vi "AODScanner1.vi"() -> ()   [LabVIEW 2014]
uses:
  AODAcq/AODAcq.lvclass
  <vilib>/DAQmx/write.llb/DAQmx Write (Analog DBL 1Chan 1Samp).vi
  Motion Stabilization/GlobalVars.vi
  <vilib>/Utility/error.llb/Error Cluster From Error Code.vi
  <vilib>/rvi/errors/niLvFpgaAdjustHostInterfaceError.vi
  <vilib>/DAQmx/read.llb/DAQmx Read (Analog Wfm 1Chan NSamp).vi
  <vilib>/rvi/interface/nirviMethod/nirviMethod.xnode
  FPGA_Control/AODRef.ctl
  FPGA Bitfiles/AodScanner_FPGATarget_AODControl(FPGA)_TyJc9yYmyGA.lvbitx
  <vilib>/rvi/interface/nirviReadWriteControl/nirviReadWriteControl.xnode
  <vilib>/FPGAPlugInAG/PXIe-7965R/niLvFpga_ReadFifo_PXIe-7965R.vi
  <vilib>/rvi/errors/niLvFpgaMergeErrorWithErrorCode.vi
  NiFpgaLv.dll
panel:
  out "globals_semaphore":T1
  out "Scan Settings Saved":T2
  out "y_scale":dbl
  out "x_scale":dbl
  out "Motion Points (Ch1)":u32
  in  "Per Cell Motion Analysis":bool
  in  "Sampling Structure":u16(ring) items=["Cube Vertices"]
  out "EventDone":bool
  in  "ForcePointScan":bool
  out "Selection":u32
  in  "ForceVolumeScan":bool
  out "Scan Settings (um) Saved":T2={"XStart"=-100, "XEnd"=100, "XNum"=250, "YStart"=-100, "YEnd"=100, "YNum"=250, "ZStart"=-30, "ZEnd"=70, "ZNum"=60}
  out "Motion FIFO":refnum<queue>
  out "Points_um":dbl[][](array[numeric])
  out "Stopped":bool
  in  "Power":dbl(slide)=2.5 min=0.0 max=5.0 step=0.1 scale=0.0..2.5
  in  "Debug":bool
  out "Number of Motion Planes":i32
  out "Motion Plane Centers":i32[][](array[numeric])
  in  "GridPoints":u16=10
  out "X-Y Motion Points":i32[][](array[numeric])
  out "Y-Z Motion Points":i32[][](array[numeric])
  out "error out":errorcluster
  out "error out 2":errorcluster
  in  "External Magnification":dbl=1.3
  in  "Matlab Server IP Address":string="10.21.16.18"
  in  "Matlab Server Shared Folder":string="c:\\temp"
  out "Histogram":dynamicdata(graph)
  out "ROIs":T3(array[cluster])
  out "Motion ROIs":T3(array[cluster])
  out "Waveform Chart":waveform(dbl)(graph)
  out "Ephys":bool
  in  "Points":i32[][](array[numeric])
  in  "Abort":bool
  out "ScanProgress":dbl(slide) scale=0.0..1.0
  in  "Simulated Motion Signal":bool
  in  "TraceElements":u32=10000
  out "Out Points":i32[][](array[numeric])
  in  "Tab Control":enum32{"Setup", "Volume", "Traces", "Motion"}(tab)
  in  "Motor Refractory Time":dbl=2.0
  in  "Motor Correction Threshold":dbl=2.0 format="%#_13g"
  in  "Motion Tracking":bool
  in  "Auto Recentering":bool
  in  "XNum":i32=100
  in  "YNum":i32=100
  in  "Onset (fraction)":dbl=0.99 format="%#_13g"
  in  "Offset (fraction)":dbl=0.01 format="%#_13g"
  in  "Post Recentering Wait (ms)":u32=1000
  in  "Store Raw":bool
  in  "Disp Volume":bool=TRUE
  in  "Save Volume":bool
  in  "Ephys Acq":bool
  in  "Motion rate (Hz)":dbl=10.0
  in  "Scan Settings (um)":T2={"XStart"=-100, "XEnd"=100, "XNum"=250, "YStart"=-100, "YEnd"=100, "YNum"=250, "ZStart"=-30, "ZEnd"=70, "ZNum"=60}
  in  "Objective":enum16{"20x Olympus"}(ring)
  in  "Scan Time (s)":dbl=300.0
  in  "Volume Reps":i32=1 min=1 max=10000
  in  "Volume Scan":bool
  in  "Points Scan":bool
  in  "Motion Channel To Analyze":i32=2 min=1 max=2
  in  "Motion Analysis":bool
  in  "Auto Motion Plane Params":T4={"Z Offset Per Box (um)"=3, "Box Size (um)"=16.0}
  in  "Mirror Ch1 Display":bool
  in  "ClearMotionCenters":bool
  in  "Point Centering":bool=TRUE
  in  "Recenter":bool caption="OK Button"
  out "Cells Selected":u32
  in  "Contrast":dbl(slide)=99.63636363636364 scale=98.0..100.0
  out "ImCh2":T5(plugin-control)
  out "ImCh1":T5(plugin-control)
  in  "Section":dbl min=0.0 max=59.0 step=1.0
  in  "Segment":bool
  out "Motion Increment":u32
  in  "Offset":dbl(slide)=0.010101010101010102 scale=0.0..1.0
  in  "ClearPoints":bool
  out "Total Motion Points":i32
  out "Number of Motion Volumes":i32
  out "Motion Ch1":T5(plugin-control)
  out "Ephys Signals":waveform(dbl)[](graph)
  in  "Baseline Offset":dbl
  in  "Decimate":bool
  in  "Spacing":dbl=100.0
  out "Traces":waveform(dbl)[](graph)
  in  "Down Rate":i32=500
  out "Motion Detection Error":bool
  in  "Enable Calibration":bool
  in  "Analyze Nth Frames":i32=1 min=1 step=1
  out "Elements in Data Queue":i32
  out "Out of Limits":bool
  in  "Position Shift Limit (Microns)":dbl=3.0 min=0.0
  out "Z1":waveform(dbl)(graph)
  out "Y1":waveform(dbl)(graph)
  out "X1":waveform(dbl)(graph)
  out "VolData":i32[][](array[numeric])
  out "Progress":dbl(slide) scale=0.0..1.0
  out "Scan Settings":T2
  in  "VolumeElements":u32=10000
  out "Recording File":path
  out "Objective Position":cluster{"X":dbl, "Y":dbl, "Z":dbl}
  out "Lens Magnification":i32=20
  out "Finished":bool
  out "Image samples remaining":u32
  out "Motion samples remaining":u32
  out "Temporal samples remaining":u32
  out "Raw samples remaining":u32
  in  "stop":bool
  out "AODAcq out":refnum<class "AODAcq.lvclass">
  out "Volume":bool
  out "Scan":bool
  in  "SweepSettings":bool
  out "Numeric":i32=299
  # "On"
  # "Off"
  # "sec"
  # "um"
  # "Motor"
  # "AOD+Motor"
  # "Off"
  # "On"
  # "Volume Resolution (points)"
  # "Behavior Pause"
  # "Off"
  # "On"
  # "Off"
  # "On"
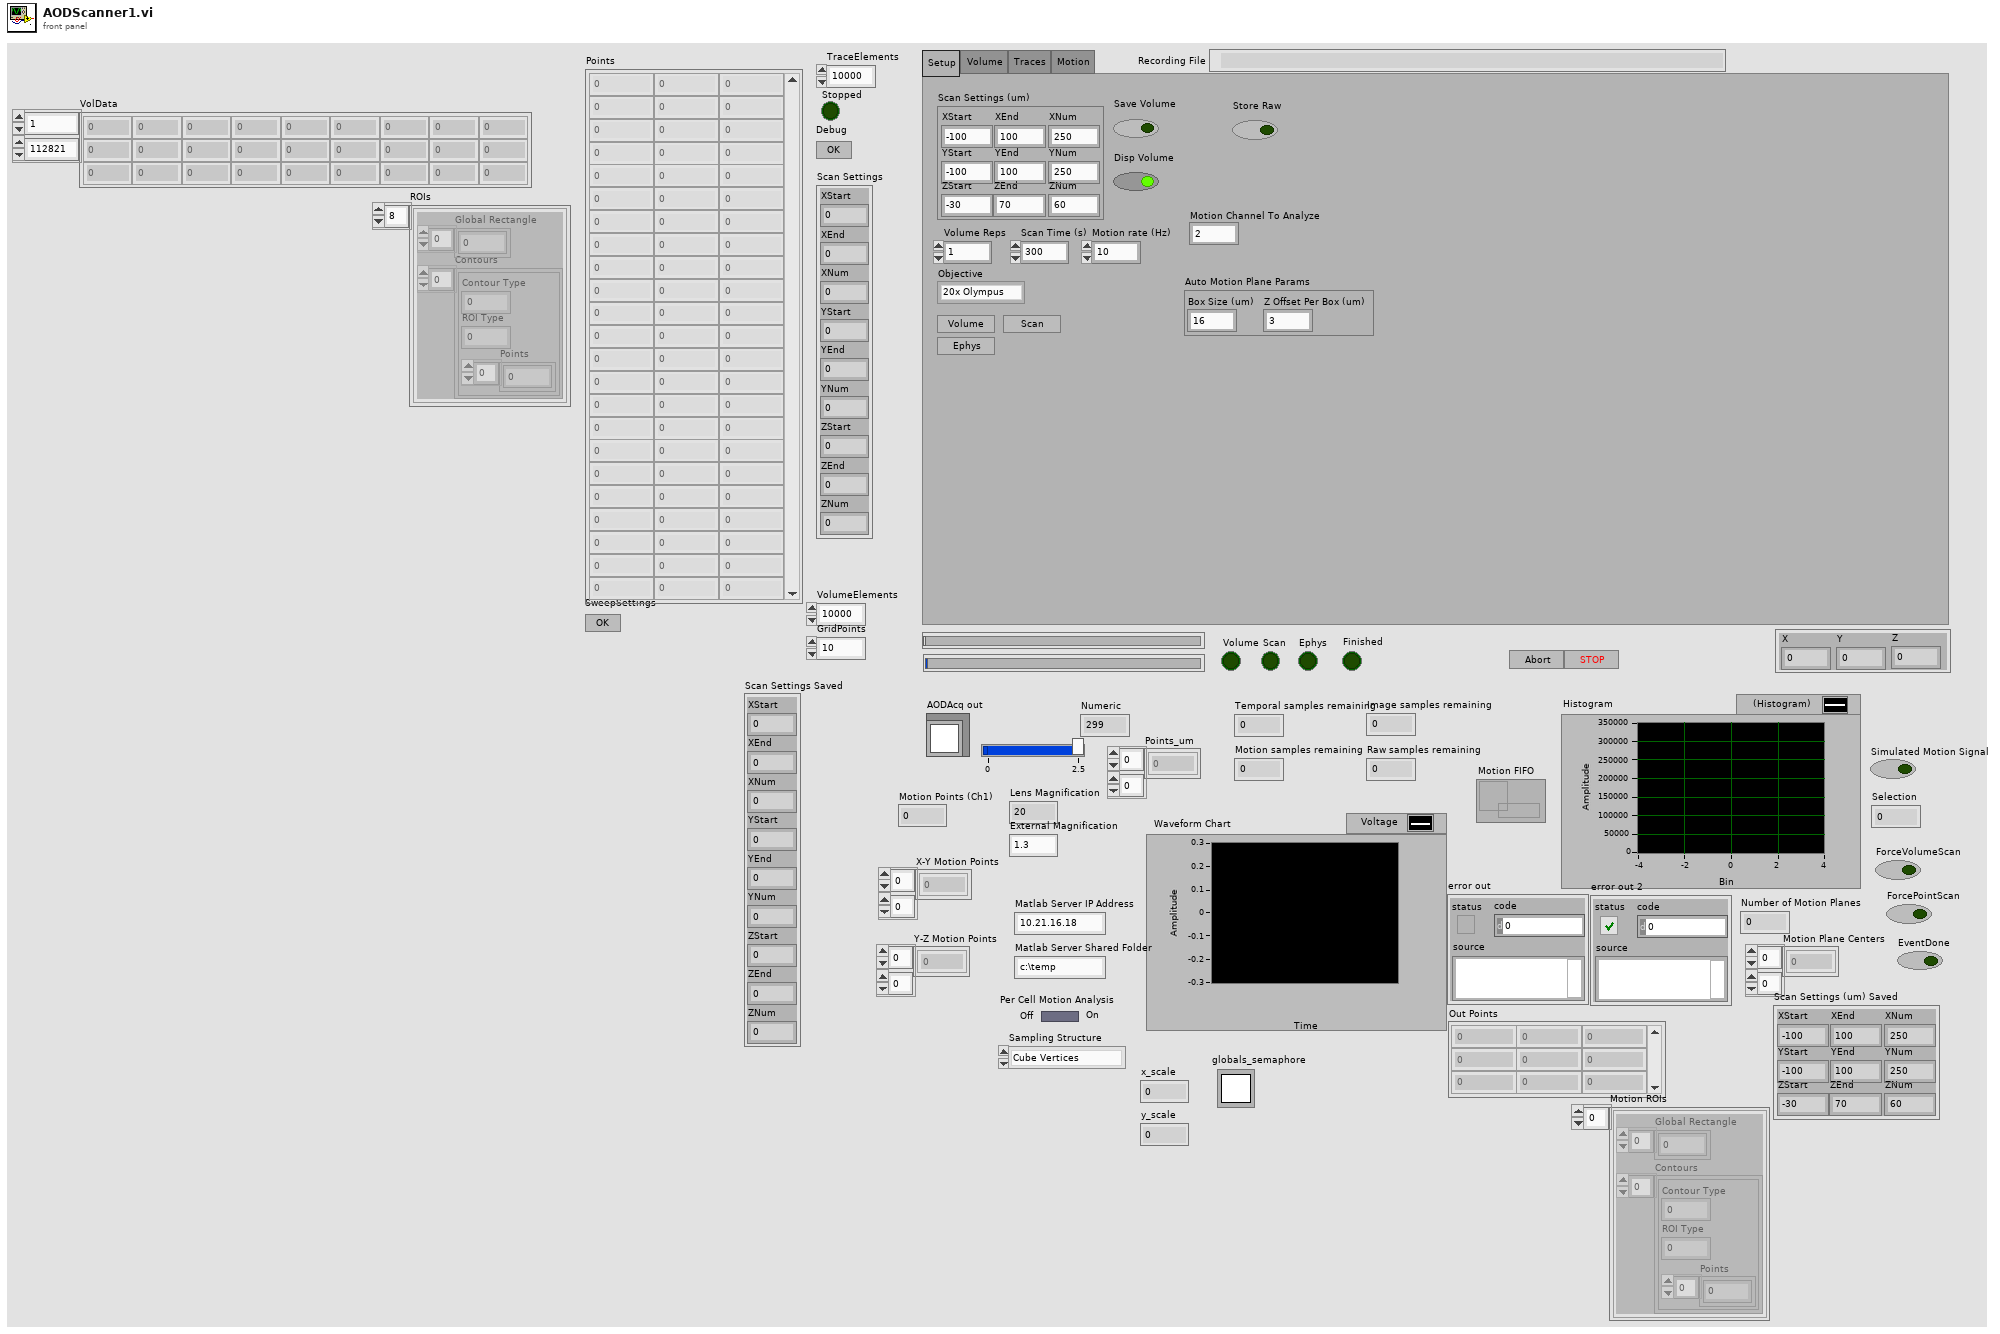
[diagram p1: front panel]
types:
  T1 = typedef "Semaphore RefNum" = refnum<k1>
  T2 = cluster{"XStart":i32, "XEnd":i32, "XNum":i32, "YStart":i32, "YEnd":i32, "YNum":i32, "ZStart":i32, "ZEnd":i32, "ZNum":i32}
  T3 = cluster{"Global Rectangle":i32[], "Contours":cluster{"Contour Type":u32, "ROI Type":u32, "Points":i32[]}[]}[]
  T4 = cluster{"Z Offset Per Box (um)":i32, "Box Size (um)":dbl}
  T5 = typedef "IMAQ Image.ctl" = refnum<image>
  T6 = cluster{"gridsize":u16, "data":i32[][], "coordinates":i32[][], "settings":i32[], "settings_um":i32[], "needsreference":bool}
  T7 = typedef "Image Type" = u32
  T8 = cluster{"Global Rectangle":i32[], "Contours":cluster{"Contour Type":u32, "ROI Type":u32, "Points":i32[]}[]}
  T9 = cluster{"queue out":refnum<queue>, "queue out":refnum<queue>, "queue out":refnum<queue>, "queue out":refnum<queue>}
  T10 = cluster{"Restarted":bool, "Enable Calibration":bool, "Position Shift Limit (Microns)":dbl, "Frame Num":dbl, "Sampling Interval":dbl, "Analyze Nth Frames":i32}
  T11 = typedef "AODRef.ctl" = refnum<k20>
  T12 = cluster{"X":waveform(dbl), "Y":waveform(dbl), "Z":waveform(dbl), "Out of Limits":bool, "Motion Detection Error":bool, "Flush Queue":i32, "Movement Signal":dbl[], "Movement Detection Time":dbl}
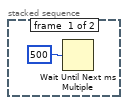
[diagram p2: hidden frame]
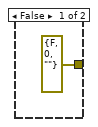
[diagram p4: hidden frame]
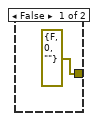
[diagram p5: hidden frame]
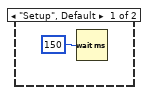
[diagram p6: hidden frame]
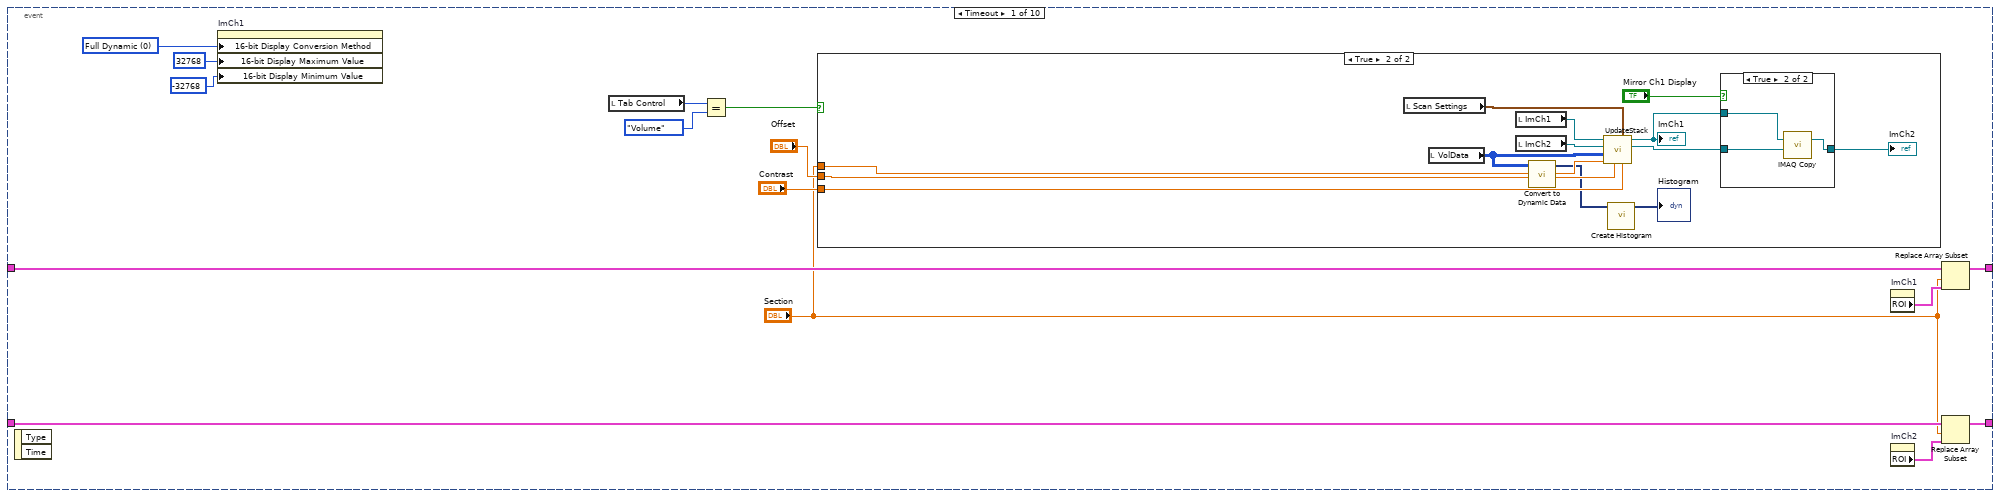
[diagram p8: hidden frame]
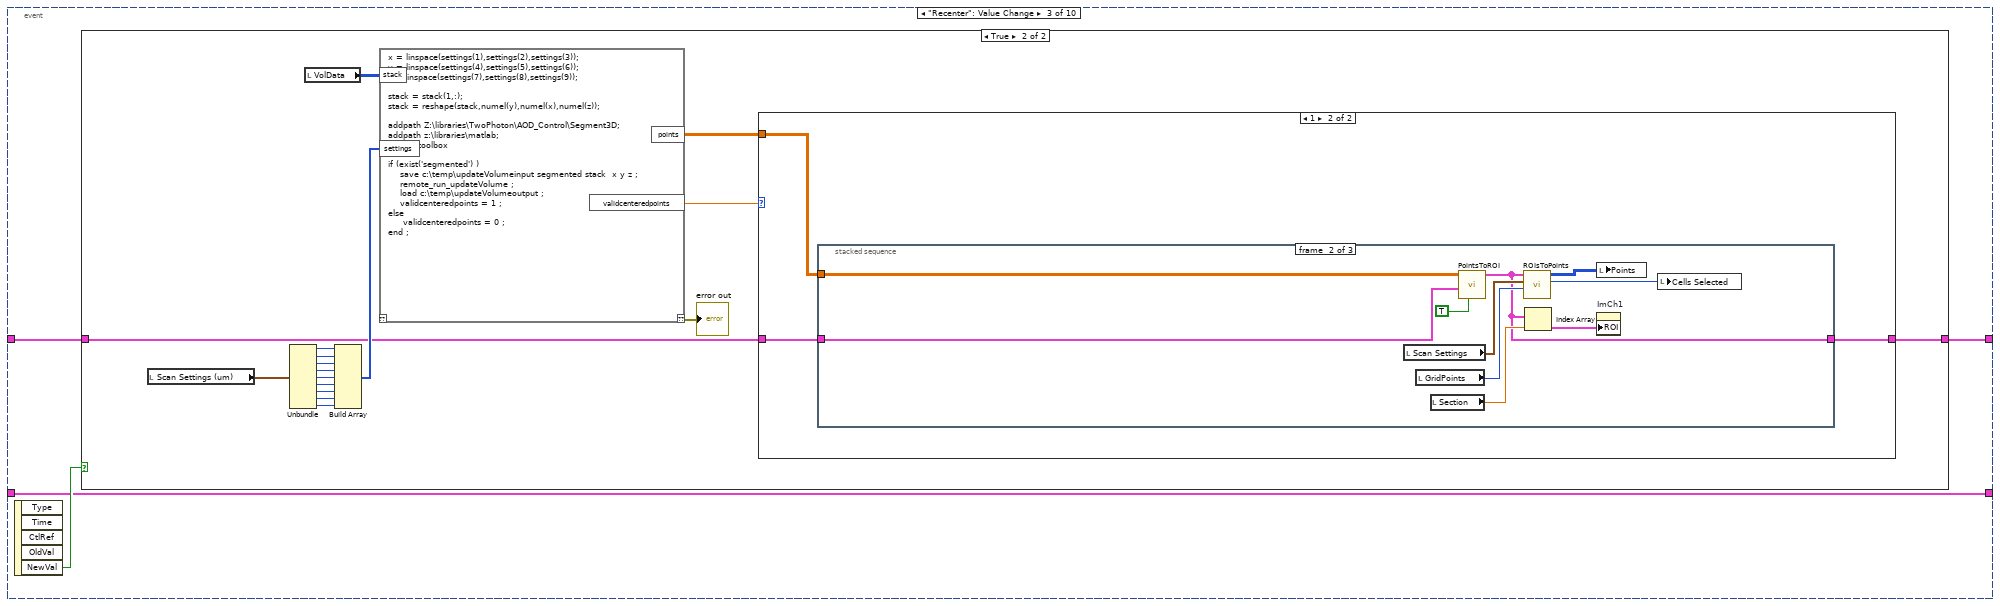
[diagram p12: hidden frame]
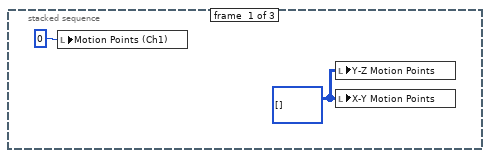
[diagram p15: hidden frame]
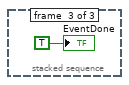
[diagram p16: hidden frame]
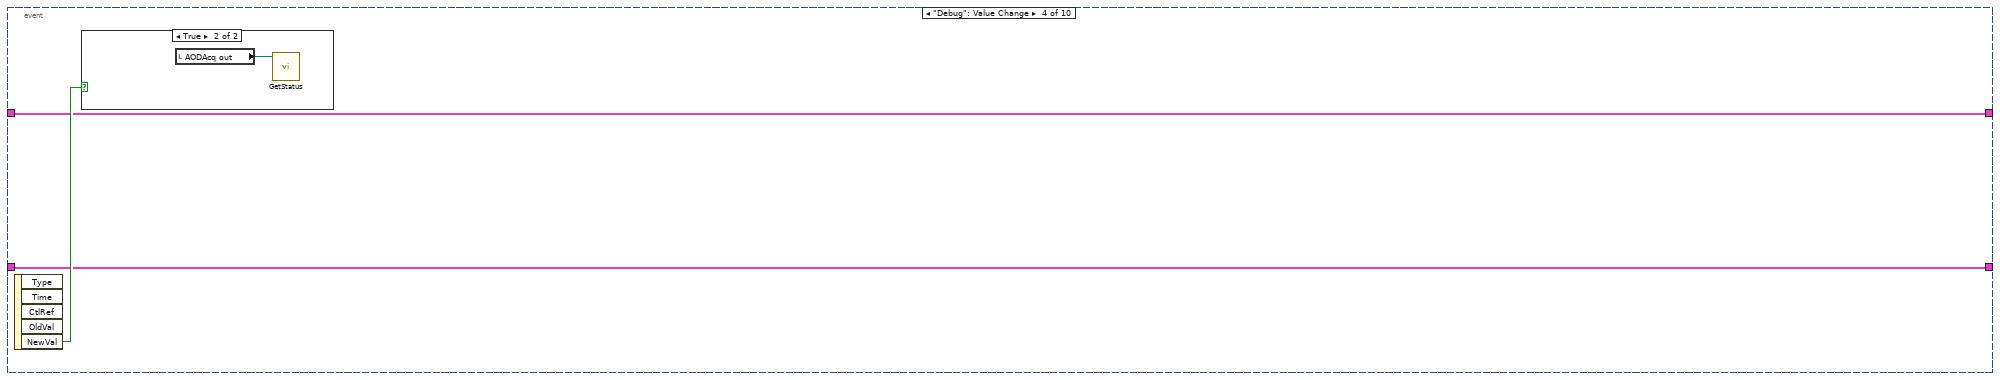
[diagram p17: hidden frame]
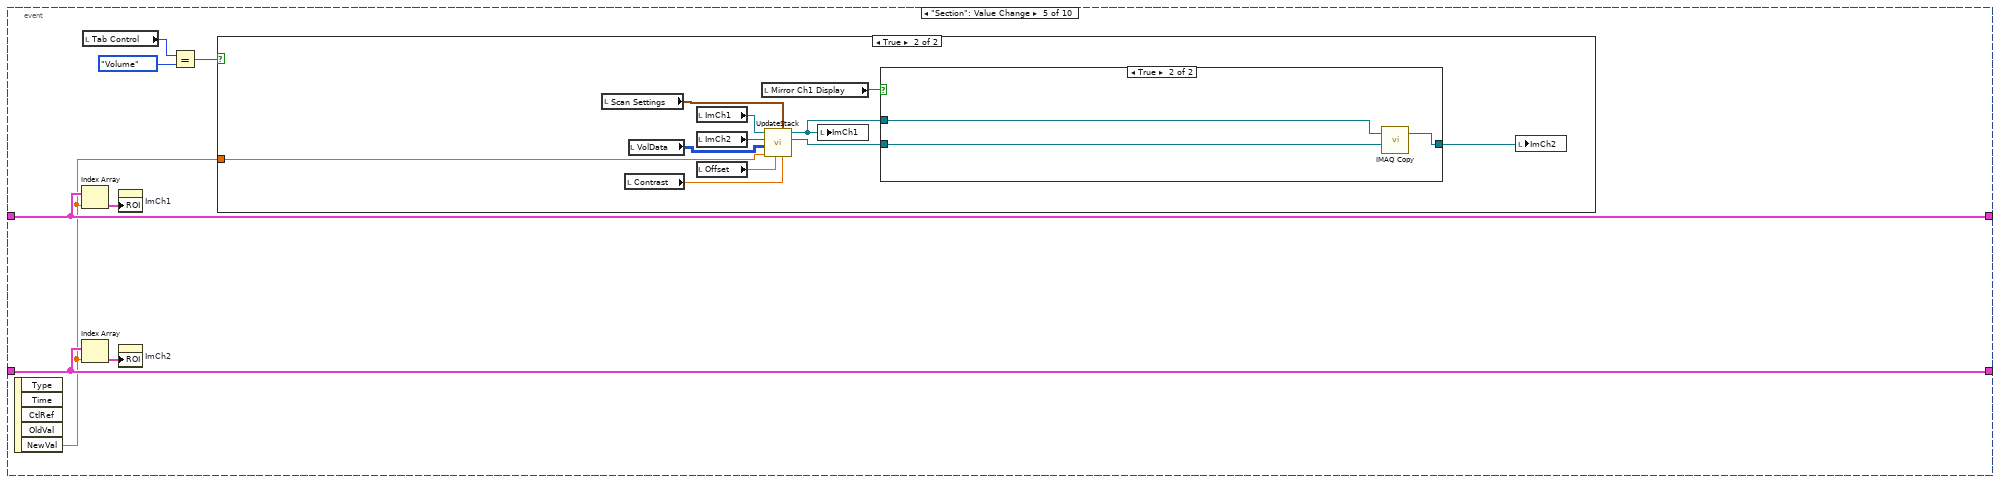
[diagram p19: hidden frame]
diagram:
  w7 = FALSE ("ForceVolumeScan")
  w24 = 100 ("max queue size (-1, unlimited)")
  w29 = T7 2 items=["Grayscale (U8)", "Grayscale (I16)", "Grayscale (SGL)", "Complex (CSG)", "RGB (U32)", "HSL (U32)", "RGB (U64)", "Grayscale (U16)"] ("Image Type")
  w5 = waveform(i32)[] []
  w39 = T7 0 items=["Grayscale (U8)", "Grayscale (I16)", "Grayscale (SGL)", "Complex (CSG)", "RGB (U32)", "HSL (U32)", "RGB (U64)", "Grayscale (U16)"] ("Image Type")
  w15 = T8 {"Global Rectangle"=[], "Contours"=[]} ("ROI")
  w49 = refnum<k21> "AOD Gain"  # DAQmx Global Channel
  n1 = local read "Scan Settings (um)"() -> (w43:T2)
  n2 = local write "ForceVolumeScan"(w7) -> ()
  n3 = local write "ForcePointScan"(w7) -> ()
  n4 = local write "Stopped"(FALSE ("Stopped")) -> ()
  n5 = local write "Stopped"(FALSE ("Stopped")) -> ()
  n6 = global write "GlobalVars.vi" "VI Open"(FALSE ("VI Open")) -> ()
  n7 = local write "Tab Control"(enum32{"Setup", "Volume", "Traces", "Motion"}."Setup" ("Tab Control")) -> ()
  n8 = Reciprocal(x="Motion rate (Hz)") -> (1/x=w17:dbl)
  n9 = global write "GlobalVars.vi" "Sampling Interval (sec)"(w17) -> ()
  n10 = call <vilib>:"DAQmx Create Task.vi"("global virtual channels"=w49) -> ("task out"=w48:refnum<k21>, "error out"=w47:errorcluster)  [unwired: 4 in, 9 out]
  n11 = call "IMAQ Create"("Image Name"="Im1", "Image Type"=w39) -> ("New Image"=w51:T5)  [unwired: 3 in, 1 out]
  n12 = call "IMAQ Create"("Image Name"="Im2", "Image Type"=w39) -> ("New Image"=w50:T5)  [unwired: 3 in, 1 out]
  n13 = Unbundle By Name(w43) -> ("ZNum"=w14:i32)
  n14 = call "IMAQ Create"("Image Name"="Mot1", "Image Type"=w29) -> ("New Image"=→"Motion Ch1":T5)  [unwired: 3 in, 1 out]
  n15 = while {
    tunnel: w48 -> [w60]
    tunnel: w47 -> [w59]
    tunnel: [w58] -> w46
    tunnel: [w57] -> w45
    stop <- w56 stop-if-true
    n16 = Wait (ms)(milliseconds to wait=u32 1000) -> ()  [unwired: 1 out]
    n17 = local read "Stopped"() -> (w56:bool)
    n18 = call-poly <vilib>:"DAQmx Write.vi"("task/channels in"=w60, "data"="Power", "error in"=w59) -> ("task out"=w58:refnum<k21>, "error out"=w57:errorcluster)  [unwired: 10 in, 1 out]
  }
  n19 = local write "ImCh1"(w51) -> ()
  n20 = local write "ImCh2"(w50) -> ()
  n21 = Obtain Queue(max queue size (-1, unlimited)=w24, element data type=waveform(i32)[] []) -> (queue out=w35:refnum<queue>)  [unwired: 3 in, 2 out]
  n22 = Obtain Queue(max queue size (-1, unlimited)=w24, element data type=waveform(dbl)[] []) -> (queue out=w36:refnum<queue>)  [unwired: 3 in, 2 out]
  n23 = Obtain Queue(max queue size (-1, unlimited)=w24, element data type=w5) -> (queue out=w34:refnum<queue>)  [unwired: 3 in, 2 out]
  n24 = Obtain Queue(element data type=w5) -> (queue out=w4:refnum<queue>)  [unwired: 4 in, 2 out]
  n25 = call <vilib>:"Obtain Semaphore Reference.vi"("name (unnamed)"="globals") -> ("error out"=w1:errorcluster, "semaphore"=w2:T1)  [unwired: 4 in, 1 out]
  "globals_semaphore" <- w2
  n26 = Obtain Queue(name (unnamed)="Motion FIFO", element data type=0) -> (queue out=w10:refnum<queue>)  [unwired: 3 in, 2 out]
  "Motion FIFO" <- w10
  n27 = Obtain Queue(max queue size (-1, unlimited)=100, name (unnamed)="MotionAnalysis", element data type=T6 {"gridsize"=0, "data"=[], "coordinates"=[], "settings"=[], "settings_um"=[], "needsreference"=FALSE}) -> (queue out=w8:refnum<queue>)  [unwired: 2 in, 2 out]
  n28 = Decrement(x=w14) -> (x-1=w38:i32)
  n29 = Initialize Array(w15, w14) -> (w42:T3)
  n30 = Initialize Array(w15, w14) -> (w13:T3)
  n31 = while {
    shift-right: [w63] -> _
    shift-left: w42 -> [w67]
    shift-right: [w62] -> _
    shift-left: w13 -> [w64]
    stop <- w65 stop-if-true
    n32 = event shown="[1] \"Segment\": Value Change" {
      selector: _ -> [_ _ _ _ _ _ _ _ _ _]
      dyn-events: _ -> [_ _ _ _ _ _ _ _ _ _]
      timeout: 200 -> [_ _ _ _ _ _ _ _ _ _]
      tunnel: w67 -> [w81 w102 w142 w181 w190 w218 w219 w232 w236 w248]
      tunnel: [w82 w101 w143 w181 w190 w215 w219 w231 w237 w248] -> w63
      tunnel: [w69 w100 w141 w180 w185 w207 w220 w228 w235 w249] -> w62
      tunnel: w64 -> [w72 w100 w141 w180 w185 w207 w225 w230 w235 w247]
      event Timeout {
        w77 = u32 0 items=["Full Dynamic", "Downshift", "Given Range", "90% Dynamic", "Given Percent Range"] ("16-bit Display Mapping:Conversion Method")
        n33 = event-data() -> ()  [unwired: 1 in, 2 out]
        n34 = property on="ImCh1" class="ImageControl"("16-bit Display Conversion Method"=w77, "16-bit Display Maximum Value"=32768 ("16-bit Display Mapping:Maximum Value"), "16-bit Display Minimum Value"=-32768 ("16-bit Display Mapping:Maximum Value")) -> ()  [unwired: 2 in, 2 out]
        n35 = local read "Tab Control"() -> (w79:enum32{"Setup", "Volume", "Traces", "Motion"})
        n36 = Equal?(x=w79, y=enum32{"Setup", "Volume", "Traces"}."Volume") -> (x = y?=w68:bool)
        n37 = case shown="True" w68 {
          tunnel: "Section" -> [_ w92]
          tunnel: "Offset" -> [_ w91]
          tunnel: "Contrast" -> [_ w90]
          frame False {
          }
          frame True {
            n38 = local read "Scan Settings"() -> (w93:T2)
            n39 = local read "VolData"() -> (w89:i32[][])
            n40 = local read "ImCh1"() -> (w95:T5)
            n41 = local read "ImCh2"() -> (w94:T5)
            n42 = call "Convert to Dynamic Data"("2D Array"=w89) -> ("Dynamic Data Type"=w88:dynamicdata)  [unwired: 3 in]
            n43 = call "UpdateStack.vi"("Contrast"=w90, "Scan Settings"=w93, "Offset"=w91, "Section"=w92, "ImData"=w89, "Im2 2"=w94, "Im1 In"=w95) -> ("Im2 Out"=w83:T5, "Im1 Out"=w85:T5)  [unwired: 3 in]
            "ImCh1" <- w85
            n44 = call "Create Histogram"("Signal"=w88) -> ("Histogram"=→"Histogram":dynamicdata)  [unwired: 9 in, 1 out]
            n45 = case shown="True" "Mirror Ch1 Display" {
              tunnel: w85 -> [_ w98]
              tunnel: [w96 w97] -> w84
              tunnel: w83 -> [w96 w99]
              frame False {
              }
              frame True {
                n46 = call "IMAQ Copy"("Image Dst"=w99, "Image Src"=w98) -> ("Image Dst Out"=w97:T5)  [unwired: 4 in, 1 out]
              }
            }
            "ImCh2" <- w84
          }
        }
        n47 = property on="ImCh1" class="ImageControl"() -> ("ROI"=w80:T8)  [unwired: 2 in, 2 out]
        n48 = property on="ImCh2" class="ImageControl"() -> ("ROI"=w71:T8)  [unwired: 2 in, 2 out]
        n49 = Replace Array Subset(array=w81, new element=w80, index="Section") -> (w82:T3)
        n50 = Replace Array Subset(array=w72, new element=w71, index="Section") -> (w69:T3)
      }
      event "Segment": Value Change {
        n51 = event-data() -> ("NewVal"=w103:bool)  [unwired: 1 in, 4 out]
        n52 = case shown="True" w103 {
          tunnel: w102 -> [w104 w122]
          tunnel: [w104 w126] -> w101
          frame False {
          }
          frame True {
            n53 = local read "Scan Settings (um)"() -> (w140:T2)
            n54 = local read "Lens Magnification"() -> (w118:i32)
            n55 = local read "Scan Settings (um)"() -> (w120:T2)
            n56 = Boolean To (0,1)(Boolean="Point Centering") -> (0, 1=w123:i16)
            n57 = Unbundle(w140) -> ("XStart"=w139:i32, "XEnd"=w138:i32, "XNum"=w137:i32, "YStart"=w136:i32, "YEnd"=w135:i32, "YNum"=w134:i32, "ZStart"=w133:i32, "ZEnd"=w132:i32, "ZNum"=w131:i32)
            n58 = Build Array(w139, w138, w137, w136, w135, w134, w133, w132, w131) -> (w112:i32[])
            n59 = To Double Precision Float(number=w123) -> (double precision float=w116:dbl)
            n60 = local read "VolData"() -> (w130:i32[][])
            n61 = Concatenate Strings("Matlab Server IP Address", "," ("string"), "Matlab Server Shared Folder") -> (w107:string)
            n62 = call "ROIsToSelCells.vi"("Scan Settings"=w120, "ROI"=w122) -> ("Points_um"=w119:dbl[][])  [unwired: 8 in, 1 out]
            n63 = Build Array (concatenate)(w118, "External Magnification", w116, w112) -> (w111:dbl[])
            n64 = script code="if (feature('numcores')>1)\n     if (~matlabpool('size') > 0)\n         matlabpool(min(feature('numcores'),12)) ;\n     end ;\nend ;\n\nlens = params(1) ;\nmagnification = params(2) ;\nenablecentering = params(3) ;\nsettings = params(4:end) ;\n\ncomma = strfind(textparams, ',') ;\nip = textparams(1:comma-1) ;\nsharedfolder = textparams(comma+1:end) ;\n\nx = linspace(settings(1),settings(2),settings(3));\ny = linspace(settings(4),settings(5),settings(6));\nz = linspace(settings(7),settings(8),settings(9));\n\nvol = vol(1,:);\nvol = reshape(vol,numel(y),numel(x),numel(z));\n\nrehash toolbox\nserver_ip = ip ;\nserver_shareddir = sharedfolder ;\n%save c:\\temp\\serverinfo server_ip ;\n\n%save c:\\temp\\segmenterinput vol x y z points lens magnification ip sharedfolder enablecentering ;\n%remote_run_segmenter ;\nseg = aod.Segmenter(vol, x, y, z, points, lens, magnification, ip, sharedfolder, enablecentering ) ;\nsegmented = SegmenterDisplay(seg) ;\n\nfilename = sprintf('%s\\\\seg.mat', sharedfolder) ;\nload(filename) ;\npoints = centered_coordinates;\npositions = points; % in microns\n\n% Need to convert points into indicies into the array\nfor i = 1:size(points,1)\n   [~,idx] = min(abs(points(i,1)-x)); points(i,1) = idx;\n   [~,idx] = min(abs(points(i,2)-y)); points(i,2) = idx;\n   [~,idx] = min(abs(points(i,3)-z)); points(i,3) = idx;\nend\noutpoints = points ;"("vol"=w130, "params"=w111, "textparams"=w107, "points"=w119) -> ("??"=→"error out 2":errorcluster, "outpoints"=w106:dbl[][], "positions"=w105:dbl[][])  [unwired: 1 in]
            n65 = call "PointsToROI.vi"("Old ROIs"=w122, "Points"=w106) -> ("ROIs"=w126:T3)  [unwired: 9 in]
            n66 = local write "Points_um"(w105) -> ()
            n67 = local read "Scan Settings"() -> (w128:T2)
            n68 = local read "GridPoints"() -> (w121:u16)
            n69 = local read "Section"() -> (w125:dbl)
            n70 = Index Array(array=w126, index=w125) -> (element=w127:T8)
            n71 = call "ROIsToPoints.vi"("GridPoints"=w121, "Scan Settings"=w128, "ROI"=w126) -> ("Number of motion points"=w109:i32, "Number of points"=w129:i32, "Points"=w108:i32[][])  [unwired: 4 in, 2 out]
            n72 = local write "Points"(w108) -> ()
            n73 = property on="ImCh1" class="ImageControl"("ROI"=w127) -> ()  [unwired: 2 in, 2 out]
            n74 = local write "Cells Selected"(w129) -> ()
            n75 = local write "Motion Points (Ch1)"(w109) -> ()
          }
        }
      }
      event "Recenter": Value Change {
        n76 = event-data() -> ("NewVal"=w144:bool)  [unwired: 1 in, 4 out]
        n77 = case shown="True" w144 {
          tunnel: [w145 w148] -> w143
          tunnel: w142 -> [w145 w149]
          frame False {
          }
          frame True {
            n78 = local read "Scan Settings (um)"() -> (w150:T2)
            n79 = Unbundle(w150) -> ("XStart"=w162:i32, "XEnd"=w161:i32, "XNum"=w160:i32, "YStart"=w159:i32, "YEnd"=w158:i32, "YNum"=w157:i32, "ZStart"=w156:i32, "ZEnd"=w155:i32, "ZNum"=w154:i32)
            n80 = local read "VolData"() -> (w152:i32[][])
            n81 = Build Array(w162, w161, w160, w159, w158, w157, w156, w155, w154) -> (w153:i32[])
            n82 = script code="x = linspace(settings(1),settings(2),settings(3));\ny = linspace(settings(4),settings(5),settings(6));\nz = linspace(settings(7),settings(8),settings(9));\n\nstack = stack(1,:);\nstack = reshape(stack,numel(y),numel(x),numel(z));\n\naddpath Z:\\libraries\\TwoPhoton\\AOD_Control\\Segment3D;\naddpath z:\\libraries\\matlab;\nrehash toolbox\n\nif (exist('segmented') )\n    save c:\\temp\\updateVolumeinput segmented stack  x y z ;\n    remote_run_updateVolume ;\n    load c:\\temp\\updateVolumeoutput ;\n    validcenteredpoints = 1 ;\nelse\n     validcenteredpoints = 0 ;\nend ;"("stack"=w152, "settings"=w153) -> ("??"=→"error out":errorcluster, "points"=w151:dbl[][], "validcenteredpoints"=w147:dbl)  [unwired: 1 in]
            n83 = case shown="1" w147 {
              tunnel: w151 -> [_ w166]
              tunnel: w149 -> [w163 w165]
              tunnel: [w163 w164] -> w148
              frame 0, Default {
              }
              frame 1 {
                n84 = stacked-sequence {
                  tunnel: w166 -> [_ w178 _]
                  tunnel: w165 -> [_ w174 _]
                  tunnel: [_ w171 _] -> w164
                  frame #0 {
                    w167 = i32[][] [] ("Points")
                    n85 = local write "Motion Points (Ch1)"(u32 0 ("Number of Motion Points")) -> ()
                    n86 = local write "Y-Z Motion Points"(w167) -> ()
                    n87 = local write "X-Y Motion Points"(w167) -> ()
                  }
                  frame #1 {
                    n88 = local read "Scan Settings"() -> (w175:T2)
                    n89 = local read "GridPoints"() -> (w176:u16)
                    n90 = local read "Section"() -> (w172:dbl)
                    n91 = call "PointsToROI.vi"("Clear Motion Planes"=TRUE, "Old ROIs"=w174, "Points"=w178) -> ("ROIs"=w171:T3)  [unwired: 8 in]
                    n92 = call "ROIsToPoints.vi"("GridPoints"=w176, "Scan Settings"=w175, "ROI"=w171) -> ("Number of points"=w177:i32, "Points"=w170:i32[][])  [unwired: 4 in, 3 out]
                    n93 = Index Array(array=w171, index=w172) -> (element=w173:T8)
                    n94 = local write "Points"(w170) -> ()
                    n95 = property on="ImCh1" class="ImageControl"("ROI"=w173) -> ()  [unwired: 2 in, 2 out]
                    n96 = local write "Cells Selected"(w177) -> ()
                  }
                  frame #2 {
                    "EventDone" <- TRUE ("EventDone")
                  }
                }
              }
            }
          }
        }
      }
      event "Debug": Value Change {
        n97 = event-data() -> ("NewVal"=w182:bool)  [unwired: 1 in, 4 out]
        n98 = case shown="True" w182 {
          frame False {
          }
          frame True {
            n99 = local read "AODAcq out"() -> (w183:refnum<class "AODAcq.lvclass">)
            n100 = call-dynamic "GetStatus.vi"("AODAcq in"=w183) -> ()  [unwired: 8 in, 3 out]
          }
        }
      }
      event "Section": Value Change {
        n101 = event-data() -> ("NewVal"=w184:dbl)  [unwired: 1 in, 4 out]
        n102 = Index Array(array=w190, index=w184) -> (element=w191:T8)
        n103 = Index Array(array=w185, index=w184) -> (element=w186:T8)
        n104 = local read "Tab Control"() -> (w189:enum32{"Setup", "Volume", "Traces", "Motion"})
        n105 = property on="ImCh1" class="ImageControl"("ROI"=w191) -> ()  [unwired: 2 in, 2 out]
        n106 = property on="ImCh2" class="ImageControl"("ROI"=w186) -> ()  [unwired: 2 in, 2 out]
        n107 = Equal?(x=w189, y=enum32{"Setup", "Volume", "Traces"}."Volume") -> (x = y?=w187:bool)
        n108 = case shown="True" w187 {
          tunnel: w184 -> [_ w199]
          frame False {
          }
          frame True {
            n109 = local read "Scan Settings"() -> (w198:T2)
            n110 = local read "Contrast"() -> (w196:dbl)
            n111 = local read "VolData"() -> (w202:i32[][])
            n112 = local read "ImCh1"() -> (w200:T5)
            n113 = local read "ImCh2"() -> (w201:T5)
            n114 = local read "Offset"() -> (w197:dbl)
            n115 = local read "Mirror Ch1 Display"() -> (w192:bool)
            n116 = call "UpdateStack.vi"("Contrast"=w196, "Scan Settings"=w198, "Offset"=w197, "Section"=w199, "ImData"=w202, "Im2 2"=w201, "Im1 In"=w200) -> ("Im2 Out"=w194:T5, "Im1 Out"=w195:T5)  [unwired: 3 in]
            n117 = local write "ImCh1"(w195) -> ()
            n118 = case shown="True" w192 {
              tunnel: w195 -> [_ w205]
              tunnel: [w203 w204] -> w193
              tunnel: w194 -> [w203 w206]
              frame False {
              }
              frame True {
                n119 = call "IMAQ Copy"("Image Dst"=w206, "Image Src"=w205) -> ("Image Dst Out"=w204:T5)  [unwired: 4 in, 1 out]
              }
            }
            n120 = local write "ImCh2"(w193) -> ()
          }
        }
      }
      event "GridPoints": Value Change; "ImCh1": Mouse Up {
        n121 = event-data() -> ()  [unwired: 1 in, 3 out]
        n122 = local read "Section"() -> (w216:dbl)
        n123 = local read "Scan Settings"() -> (w214:T2)
        n124 = property on="ImCh1" class="ImageControl"() -> ("ROI"=w217:T8)  [unwired: 2 in, 2 out]
        n125 = Replace Array Subset(array=w218, new element=w217, index=w216) -> (w215:T3)
        n126 = call "ROIsToPoints.vi"("GridPoints"="GridPoints", "Scan Settings"=w214, "ROI"=w215) -> ("X-Y Motion Points"=→"X-Y Motion Points":i32[][], "Number of motion points"=→"Motion Points (Ch1)":i32, "Number of points"=→"Cells Selected":i32, "Points"=w212:i32[][], "Y-Z Motion Points"=→"Y-Z Motion Points":i32[][])  [unwired: 4 in]
        n127 = local write "Points"(w212) -> ()
      }
      event "ImCh2": Mouse Up {
        n128 = event-data() -> ()  [unwired: 1 in, 3 out]
        n129 = local read "Section"() -> (w226:dbl)
        n130 = local read "Scan Settings"() -> (w224:T2)
        n131 = property on="ImCh2" class="ImageControl"() -> ("ROI"=w227:T8)  [unwired: 2 in, 2 out]
        n132 = local read "GridPoints"() -> (w223:u16)
        n133 = Replace Array Subset(array=w225, new element=w227, index=w226) -> (w220:T3)
        n134 = call "ROIsToPoints.vi"("GridPoints"=w223, "Scan Settings"=w224, "ROI"=w220) -> ("Number of points"=→"Number of Motion Planes":i32, "Points"=→"Motion Plane Centers":i32[][])  [unwired: 4 in, 3 out]
      }
      event "Scan Settings (um).ZNum": Value Change {
        n135 = event-data() -> ("NewVal"=w229:i32)  [unwired: 1 in, 4 out]
        n136 = Decrement(x=w229) -> (x-1=w233:i32)
        n137 = property on="Section" class="DigNum (strict)"("Maximum"=w233, "Minimum"=0.0 ("Data Entry Limits:Minimum")) -> ()  [unwired: 2 in, 2 out]
        n138 = Reshape Array(w232, w229) -> (w231:T3)
        n139 = Reshape Array(w230, w229) -> (w228:T3)
      }
      event "ClearPoints": Value Change {
        n140 = event-data() -> ("NewVal"=w238:bool)  [unwired: 1 in, 4 out]
        n141 = case shown="True" w238 {
          tunnel: [w239 w246] -> w237
          tunnel: w236 -> [w239 _]
          frame False {
          }
          frame True {
            w240 = u32 0 ("Number of Motion Points")
            w241 = i32[][] [] ("Points")
            w245 = T8 {"Global Rectangle"=[], "Contours"=[]} ("ROI")
            n142 = local write "Points"(w241) -> ()
            n143 = local write "Points_um"(dbl[][] [] ("Points_um")) -> ()
            n144 = local write "Cells Selected"(w240) -> ()
            n145 = local write "Motion Points (Ch1)"(w240) -> ()
            n146 = local read "Scan Settings"() -> (w244:T2)
            n147 = local write "Y-Z Motion Points"(w241) -> ()
            n148 = local write "X-Y Motion Points"(w241) -> ()
            n149 = property on="ImCh1" class="ImageControl"("ROI"=w245) -> ()  [unwired: 2 in, 2 out]
            n150 = Unbundle By Name(w244) -> ("ZNum"=w243:i32)
            n151 = Initialize Array(w245, w243) -> (w246:T3)
          }
        }
      }
      event "ClearMotionCenters": Value Change {
        n152 = event-data() -> ("NewVal"=w250:bool)  [unwired: 1 in, 4 out]
        n153 = case shown="True" w250 {
          tunnel: [w251 w252] -> w249
          tunnel: w247 -> [w251 _]
          frame False {
          }
          frame True {
            w253 = T8 {"Global Rectangle"=[], "Contours"=[]} ("ROI")
            n154 = local read "Scan Settings"() -> (w255:T2)
            n155 = property on="ImCh2" class="ImageControl"("ROI"=w253) -> ()  [unwired: 2 in, 2 out]
            n156 = Unbundle By Name(w255) -> ("ZNum"=w254:i32)
            n157 = Initialize Array(w253, w254) -> (w252:T3)
          }
        }
      }
    }
    "ROIs" <- w63
    "Motion ROIs" <- w62
    n158 = local read "Stopped"() -> (w65:bool)
  }
  n159 = global write "GlobalVars.vi" "MotionAnalysis"(w8) -> ()
  n160 = property on="Section" class="DigNum (strict)"("Increment"=1.0 ("Data Entry Limits:Increment"), "Maximum"=w38, "Minimum"=0.0 ("Data Entry Limits:Minimum")) -> ()  [unwired: 2 in, 2 out]
  n161 = Bundle("queue out"=w35, "queue out"=w36, "queue out"=w34, "queue out"=w4) -> (w33:T9)  [unwired: 1 in]
  n162 = call-dynamic "FpgaInit.vi"("AODAcq in"=refnum<class "AODAcq.lvclass"> refnum ("AODAcq.lvclass")) -> ("error out"=w27:errorcluster, "AODAcq out"=w26:refnum<class "AODAcq.lvclass">)  [unwired: 9 in]
  n163 = call <vilib>:"DAQmx Clear Task.vi"("task in"=w46, "error in"=w45) -> ()  [unwired: 13 in, 1 out]
  n164 = Unbundle(w33) -> ("queue out"=w32:refnum<queue>)  [unwired: 3 out]
  n165 = while {
    shift-right: [w265] -> _
    shift-left: w26 -> [w295]
    tunnel: w33 -> [w284]
    tunnel: w27 -> [w294]
    tunnel: ["stop"] -> w18
    tunnel: w8 -> [w286]
    tunnel: w10 -> [w285]
    tunnel: w2 -> [w257]
    tunnel: w1 -> [w256]
    i -> [w287]
    stop <- "stop" stop-if-true
    n166 = call <vilib>:"Acquire Semaphore.vi"("error in (no error)"=w256, "semaphore"=w257) -> ("error out"=w260:errorcluster, "semaphore out"=w261:T1)  [unwired: 3 in, 1 out]
    n167 = Unbundle(w284) -> ("queue out"=w283:refnum<queue>, "queue out"=w282:refnum<queue>, "queue out"=w281:refnum<queue>, "queue out"=w267:refnum<queue>)
    n168 = Flush Queue(queue=w283) -> ()  [unwired: 1 in, 3 out]
    n169 = Flush Queue(queue=w282) -> ()  [unwired: 1 in, 3 out]
    n170 = Flush Queue(queue=w281) -> ()  [unwired: 1 in, 3 out]
    n171 = Flush Queue(queue=w267) -> ()  [unwired: 1 in, 3 out]
    n172 = case shown="True" TRUE {
      tunnel: w261 -> [w297 w299]
      tunnel: w260 -> [w296 w298]
      tunnel: [w297 w299] -> w259
      tunnel: [w296 w298] -> w258
      frame False {
      }
      frame True {
        n173 = Get Date/Time In Seconds() -> (seconds since 1Jan1904=w304:timestamp)
        n174 = Initialize Array(0.0 ("element"), 3 ("dimension size")) -> (w300:dbl[])
        n175 = global write "GlobalVars.vi" "MovementSignal"(w300) -> ()
        n176 = shared-variable "My Computer\\SutterShared.lvlib\\TargetPosition"(w300) -> ()  [unwired: 1 in, 1 out]
        n177 = To Double Precision Float(number=w304) -> (double precision float=w303:dbl)
        n178 = global write "GlobalVars.vi" "TargetPositionUpdateTime"(w303) -> ()
        n179 = global write "GlobalVars.vi" "MovementDetectionTime"(w303) -> ()
      }
    }
    n180 = Or(x="ForcePointScan", y="Points Scan") -> (x .or. y?=w275:bool)
    n181 = Or(x="ForceVolumeScan", y="Volume Scan") -> (x .or. y?=w279:bool)
    n182 = Build Array(w279, w275, "SweepSettings", "Ephys Acq") -> (w293:bool[])
    n183 = Boolean Array To Number(Boolean array=w293) -> (number=w292:u32)
    "Selection" <- w292
    n184 = case shown="2" w292 {
      tunnel: w295 -> [w410 w437 w517 w899 w922]
      tunnel: w294 -> [w417 w436 w560 w898 _]
      tunnel: [w410 w449 w509 w903 w922] -> w266
      tunnel: [w417 w446 w533 w902 w921] -> w264
      tunnel: w284 -> [w414 w450 w576 _ w924]
      tunnel: "Save Volume" -> [_ w445 _ _ _]
      tunnel: w286 -> [_ _ w507 _ _]
      tunnel: w285 -> [_ _ w545 _ _]
      frame 0, Default {
        n185 = call-dynamic "Read FPGA VI Reference.vi"("AODAcq in"=w410) -> ("FPGA VI Reference"=w401:T11)  [unwired: 8 in, 2 out]
        n186 = Unbundle(w414) -> ("queue out"=w413:refnum<queue>, "queue out"=w412:refnum<queue>, "queue out"=w411:refnum<queue>)  [unwired: 1 out]
        n187 = shared-variable "My Computer\\AODAcq.lvclass\\ReadFraction"(0.0 ("ReadFraction")) -> ()  [unwired: 1 in, 1 out]
        n188 = shared-variable "My Computer\\BehaviorShared.lvlib\\PauseBehavior"(FALSE ("PauseBehavior")) -> ()  [unwired: 1 in, 1 out]
        n189 = Wait (ms)(milliseconds to wait=u32 50) -> ()  [unwired: 1 out]
        n190 = Flush Queue(queue=w413) -> ()  [unwired: 1 in, 3 out]
        n191 = Flush Queue(queue=w412) -> ()  [unwired: 1 in, 3 out]
        n192 = Flush Queue(queue=w411) -> ()  [unwired: 1 in, 3 out]
        n193 = xnode "Invoke Method"("FPGA VI Reference In"=w401, "Number of Elements"=u32 0) -> ("Elements Remaining"=→"Motion samples remaining":u32)  [unwired: 2 in, 3 out]
        n194 = xnode "Invoke Method"("FPGA VI Reference In"=w401, "Number of Elements"=u32 0) -> ("Elements Remaining"=→"Image samples remaining":u32)  [unwired: 2 in, 3 out]
        n195 = xnode "Invoke Method"("FPGA VI Reference In"=w401, "Number of Elements"=u32 0) -> ("Elements Remaining"=→"Raw samples remaining":u32)  [unwired: 2 in, 3 out]
        n196 = xnode "Invoke Method"("FPGA VI Reference In"=w401, "Number of Elements"=u32 0) -> ("Elements Remaining"=→"Temporal samples remaining":u32)  [unwired: 2 in, 3 out]
        "Finished" <- FALSE ("Finished")
      }
      frame 1 {
        # "Volume imaging mode"
        n197 = local write "Volume Scan"(FALSE ("Volume")) -> ()
        n198 = local write "Tab Control"(enum32{"Setup", "Volume", "Traces"}."Volume" ("Tab Control")) -> ()
        n199 = case shown="\"20x Olympus\", Default" "Objective" {
          tunnel: [T2 {"XStart"=1460000, "XEnd"=1460000, "XNum"=1, "YStart"=1460000, "YEnd"=1460000, "YNum"=1, "ZStart"=700, "ZEnd"=700, "ZNum"=1} ("y")] -> w465
          tunnel: [20] -> w422
          frame "20x Olympus", Default {
          }
        }
        "Lens Magnification" <- w422
        n200 = call-dynamic "Init.vi"("error in (no error)"=w436, "Channel"=i16 3, "AODAcq in"=w437) -> ("error out"=w435:errorcluster, "AODAcq out"=w434:refnum<class "AODAcq.lvclass">)  [unwired: 7 in]
        n201 = call "GetObjectivePosition.vi"() -> ("output cluster"=w423:cluster{"X":dbl, "Y":dbl, "Z":dbl})  [unwired: 8 in, 3 out]
        "Objective Position" <- w423
        n202 = call-dynamic "Reset.vi"("error in (no error)"=w435, "AODAcq in"=w434) -> ("error out"=w426:errorcluster, "AODAcq out"=w427:refnum<class "AODAcq.lvclass">)  [unwired: 8 in]
        n203 = local read "ForceVolumeScan"() -> (w419:bool)
        n204 = Unbundle By Name("Scan Settings (um)") -> ("XNum"=w467:i32, "YNum"=w466:i32, "ZNum"=w431:i32)
        n205 = call-dynamic "Write Object Position.vi"("error in (no error)"=w426, "Object Position"=w423, "AODAcq in"=w427) -> ("error out"=w424:errorcluster, "AODAcq out"=w425:refnum<class "AODAcq.lvclass">)  [unwired: 7 in]
        n206 = Multiply(x=w465, y="Scan Settings (um)") -> (x*y=w420:T2)
        "Scan Settings" <- w420
        n207 = case shown="False" w419 {
          tunnel: "Scan Settings (um)" -> [w471 _]
          tunnel: w420 -> [w470 _]
          frame False {
            "Scan Settings (um) Saved" <- w471
            "Scan Settings Saved" <- w470
          }
          frame True {
          }
        }
        n208 = call-dynamic "Configure Volume.vi"("Save"=w445, "error in (no error)"=w424, "NumReps"="Volume Reps", "Scan Settings"=w420, "AODAcq in"=w425) -> ("error out"=w453:errorcluster, "AODAcq out"=w454:refnum<class "AODAcq.lvclass">)  [unwired: 5 in]
        n209 = Select(t=w431, s="Disp Volume", f=u32 1) -> (s? t:f=w430:u32)
        n210 = Compound Arithmetic op=MULTIPLY(w467, w466, w430) -> (w428:u32)
        n211 = call-dynamic "Start.vi"("error in (no error)"=w453, "AODAcq in"=w454) -> ("error out"=w441:errorcluster, "AODAcq out"=w443:refnum<class "AODAcq.lvclass">)  [unwired: 8 in]
        n212 = call-dynamic "Read Recording File.vi"("error in (no error)"=w441, "AcquistionObject in"=w443) -> ("error out"=w440:errorcluster, "Recording File"=→"Recording File":path, "AcquistionObject out"=w442:refnum<class "AODAcq.lvclass">)  [unwired: 7 in]
        n213 = call-dynamic "Read FPGA VI Reference.vi"("error in (no error)"=w440, "AODAcq in"=w442) -> ("error out"=w451:errorcluster, "FPGA VI Reference"=w457:T11, "AODAcq out"=w452:refnum<class "AODAcq.lvclass">)  [unwired: 7 in]
        n214 = Unbundle(w450) -> ("queue out"=w458:refnum<queue>, "queue out"=w455:refnum<queue>)  [unwired: 2 out]
        n215 = Initialize Array(0, 2 ("dimension size"), w428) -> (w464:i32[][])
        n216 = call-dynamic "Read Loop.vi"("error in (no error)"=w451, "ReadElements"="VolumeElements", "Queues"=w450, "AODAcq in"=w452) -> ("error out"=w447:errorcluster, "AODAcq out"=w448:refnum<class "AODAcq.lvclass">)  [unwired: 6 in]
        n217 = while {
          tunnel: w458 -> [w488]
          shift-right: [w474] -> _
          shift-left: w464 -> [w476]
          shift-right: [w485] -> _
          shift-left: 0 -> [w486]
          tunnel: w428 -> [w484]
          tunnel: 1000 ("timeout in ms (-1)") -> [w483]
          tunnel: w457 -> [w480]
          tunnel: w455 -> [w478]
          stop <- w481 stop-if-true
          n218 = Flush Queue(queue=w478) -> ()  [unwired: 1 in, 3 out]
          n219 = local read "Abort"() -> (w477:bool)
          n220 = xnode "Read/Write Control"("FPGA VI Reference In"=w480, "Control.Abort"=w477) -> ()  [unwired: 1 in, 2 out]
          n221 = Dequeue Element(queue=w488, timeout in ms (-1)=w483) -> (element=w487:waveform(i32)[], timed out?=w475:bool)  [unwired: 1 in, 2 out]
          n222 = shared-variable "My Computer\\AODAcq.lvclass\\ScanFraction"() -> (w479:dbl)  [unwired: 1 in, 1 out]
          n223 = shared-variable "My Computer\\AODAcq.lvclass\\ReadFraction"() -> (→"Progress":dbl)  [unwired: 1 in, 1 out]
          n224 = case shown="True" w475 {
            tunnel: w476 -> [w494 w503]
            tunnel: w487 -> [w493 _]
            tunnel: w486 -> [w492 w502]
            tunnel: [w491 w502] -> w485
            tunnel: [w490 w503] -> w474
            tunnel: w484 -> [w489 _]
            tunnel: [_ w501] -> w481
            frame False {
              n225 = for {
                tunnel: w494 -> [w498] mode=indexing
                tunnel: w493 -> [w500] mode=indexing
                tunnel: [w499] -> w490 mode=indexing
                tunnel: w492 -> [w496]
                tunnel: [w497] -> w491
                tunnel: w489 -> [_]
                n226 = Unbundle By Name(w500) -> ("Y"=w495:i32[])
                n227 = call "WraparoundUpdate.vi"("Data"=w495, "Location"=w496, "Accumulator"=w498) -> ("NewLocation"=w497:u32, "Accumulated"=w499:i32[])  [unwired: 7 in]
              }
            }
            frame True {
              n228 = local read "Finished"() -> (w501:bool)
            }
          }
          "VolData" <- w474
          n229 = local write "ScanProgress"(w479) -> ()
          n230 = global write "GlobalVars.vi" "VolumeData"(w474) -> ()
        }
        n231 = call-dynamic "Stop.vi"("error in (no error)"=w447, "AODAcq in"=w448) -> ("error out"=w446:errorcluster, "AODAcq out"=w449:refnum<class "AODAcq.lvclass">)  [unwired: 8 in]
        n232 = flat-sequence {
          tunnel: w447 -> [_]
          tunnel: [FALSE] -> w444
          frame #0 {
            n233 = local write "Finished"(TRUE ("Finished")) -> ()
          }
        }
        n234 = local write "Save Volume"(w444) -> ()
      }
      frame 2 {
        w513 = 3 ("dimension size")
        w514 = 0.0 ("element")
        w561 = i16 3  # Timestamp Timer Channel
        w538 = 300 ("timeout in ms (-1)")
        # "Point imaging mode"
        n235 = Flush Queue(queue=w545) -> (queue out=w544:refnum<queue>)  [unwired: 1 in, 2 out]
        n236 = global write "GlobalVars.vi" "Scanning"(TRUE ("Scanning")) -> ()
        n237 = local write "Points Scan"(FALSE ("Scan")) -> ()
        n238 = local write "Tab Control"(enum32{"Setup", "Volume", "Traces"}."Traces" ("Tab Control")) -> ()
        n239 = call-dynamic "Init.vi"("error in (no error)"=w560, "Channel"=w561, "AODAcq in"=w517) -> ("error out"=w556:errorcluster, "AODAcq out"=w553:refnum<class "AODAcq.lvclass">)  [unwired: 7 in]
        n240 = call "GetObjectivePosition.vi"() -> ("output cluster"=w552:cluster{"X":dbl, "Y":dbl, "Z":dbl})  [unwired: 8 in, 3 out]
        n241 = local read "Simulated Motion Signal"() -> (w534:bool)
        n242 = local read "Scan Settings (um)"() -> (w526:T2)
        n243 = local write "Objective Position"(w552) -> ()
        n244 = local read "Cells Selected"() -> (w546:u32)
        n245 = call-dynamic "Write Object Position.vi"("error in (no error)"=w556, "Object Position"=w552, "AODAcq in"=w553) -> ("error out"=w555:errorcluster, "AODAcq out"=w554:refnum<class "AODAcq.lvclass">)  [unwired: 7 in]
        n246 = local read "Scan Settings"() -> (w527:T2)
        n247 = call-dynamic "Reset.vi"("error in (no error)"=w555, "AODAcq in"=w554) -> ("error out"=w583:errorcluster, "AODAcq out"=w550:refnum<class "AODAcq.lvclass">)  [unwired: 8 in]
        n248 = case shown="True" w534 {
          tunnel: [dbl[][] [] w714] -> w542
          tunnel: [dbl[][] [] w712] -> w536
          tunnel: w527 -> [_ w718]
          tunnel: w526 -> [_ w717]
          frame False {
          }
          frame True {
            # "The volume is 250x250x60, so the scan settings are set to this"
            n249 = Cluster To Array(cluster=w718) -> (array=w716:i32[])
            n250 = Cluster To Array(cluster=w717) -> (array=w715:i32[])
            n251 = call "ReadTestData.vi"("settings_um"=w715, "settings_aod"=w716) -> ("coordinates"=w712:dbl[][], "linearvolume"=w713:dbl[][], "testdata"=w714:dbl[][])  [unwired: 7 in]
            n252 = global write "GlobalVars.vi" "VolumeData"(w713) -> ()
          }
        }
        n253 = local read "Motion Points (Ch1)"() -> (w521:u32)
        n254 = local read "Motion rate (Hz)"() -> (w528:dbl)
        n255 = local read "Motion ROIs"() -> (w531:T3)
        n256 = local read "GridPoints"() -> (w529:u16)
        n257 = call-dynamic "ConfigurePerCellMotionAnalysis.vi"("Scan Settings (um)"=w526, "Points Selected"=w546, "Scan Settings"=w527, "Sampling Structure"="Sampling Structure", "Per Cell Motion Analysis"="Per Cell Motion Analysis", "In Points"="Points", "AODAcq in"=w550) -> ("Additional Points"=w548:i32, "Out Points"=w530:i32[][])  [unwired: 1 in, 2 out]
        n258 = call "AutoConfigureAdditionalMotionPlanes.vi"("Motion ROIs"=w531, "In Points"=w530, "Grid Points"=w529, "Motion Rate (Hz)"=w528, "Number of Motion Points"=w521, "Scan Settings"=w527, "Plane Params"="Auto Motion Plane Params", "Scan Settings (um)"=w526) -> ("X-Y Motion Points"=w519:i32[][], "Y-Z Motion Points"=w525:i32[][], "Out Points"=w524:i32[][], "Total Motion Points"=w523:i32, "Number of Motion Volumes"=→"Number of Motion Volumes":i32, "Motion Increment"=w522:i32)  [unwired: 4 in, 2 out]
        "Out Points" <- w524
        "Total Motion Points" <- w523
        n259 = case shown="False" "Per Cell Motion Analysis" {
          tunnel: w546 -> [w770 w774]
          tunnel: w548 -> [_ w773]
          tunnel: [w770 w771] -> w541
          frame False {
          }
          frame True {
            n260 = Multiply(x=w774, y=w773) -> (x*y=w772:u32)
            n261 = Add(x=w774, y=w772) -> (x+y=w771:u32)
          }
        }
        n262 = local read "GridPoints"() -> (w571:u16)
        n263 = Quotient & Remainder(x=w523, y=w571) -> (floor(x/y)=w572:i32)  [unwired: 1 out]
        n264 = local write "X-Y Motion Points"(w519) -> ()
        n265 = local write "Motion Increment"(w522) -> ()
        n266 = local write "Y-Z Motion Points"(w525) -> ()
        n267 = Multiply(x="Scan Time (s)", y=50000.0) -> (x*y=w580:dbl)
        n268 = Decrement(x=w522) -> (x-1=w567:i32)
        n269 = Divide(x=w567, y=w522) -> (x/y=w566:dbl)
        n270 = Divide(x=w580, y=w541) -> (x/y=w569:dbl)
        n271 = Quotient & Remainder(x="TraceElements", y=w541) -> (floor(x/y)=w539:u32)  [unwired: 1 out]
        n272 = Unbundle(w576) -> ("queue out"=w540:refnum<queue>, "queue out"=w573:refnum<queue>)  [unwired: 2 out]
        n273 = Multiply(x=w566, y=w569) -> (x*y=w568:dbl)
        n274 = Multiply(x=w541, y=w539) -> (x*y=w577:u32)
        n275 = Initialize Array "Cumulative Motor Motion Signal"(w514, w513) -> (w516:dbl[])
        n276 = while {
          tunnel: w541 -> [w724]
          tunnel: w540 -> [w723]
          tunnel: w539 -> [w722]
          tunnel: w538 -> [w721]
          tunnel: 0 -> [w720]
          stop <- w719 continue-if-true
          n277 = Dequeue Element(queue=w723, timeout in ms (-1)=w721) -> (element=w726:waveform(i32)[])  [unwired: 1 in, 3 out]
          n278 = Divide(x=50000, y=w724) -> (x/y=w731:dbl)
          n279 = Divide(x=w731, y="Down Rate") -> (x/y=w733:dbl)
          n280 = Round To Nearest(number=w733) -> (nearest integer value=w729:dbl)
          n281 = In Range and Coerce(upper limit=w722, x=w729, lower limit=1.0) -> (coerced(x)=w727:dbl)  [unwired: 1 out]
          n282 = case shown="\"Traces\"" "Tab Control" {
            tunnel: w724 -> [_ w750]
            tunnel: w726 -> [_ w756]
            tunnel: w727 -> [_ w753]
            tunnel: w720 -> [_ w734]
            frame Default {
            }
            frame "Traces" {
              n283 = Index Array(array=w756, index=0) -> (element=w737:waveform(i32))
              n284 = Add(x=w737, y="Baseline Offset") -> (x+y=w735:waveform(dbl))
              n285 = Unbundle By Name(w735) -> ("dt"=w758:dbl, "Y"=w755:dbl[])
              n286 = Multiply(x=w750, y=w758) -> (x*y=w757:dbl)
              n287 = Array Size(array=w755) -> (size(s)=w745:i32)
              n288 = Divide(x=w745, y=w750) -> (x/y=w749:dbl)
              n289 = feedback #1(w734) -> (w744:i32)
              n290 = Add(x=w745, y=w744) -> (x+y=w740:i32)
              n291 = feedback-in #1(w740) -> ()
              n292 = Reshape Array(w755, w749, w750) -> (w748:dbl[][])
              n293 = Less?(x=w740, y=50000) -> (x < y?=w738:bool)
              n294 = Transpose 2D Array(2D array=w748) -> (transposed array=w747:dbl[][])
              n295 = for {
                tunnel: w757 -> [w769]
                tunnel: w735 -> [w768]
                tunnel: [w767] -> w752 mode=indexing
                tunnel: w747 -> [w766] mode=indexing
                n296 = Bundle By Name(cluster=w768, "dt"=w769, "Y"=w766) -> (w767:waveform(dbl))
              }
              n297 = Select(t=1.0, s=w738, f=0.001 ("Baseline Rate")) -> (s? t:f=w741:dbl)
              n298 = case shown="True" "Decimate" {
                tunnel: "Spacing" -> [_ w765]
                tunnel: w753 -> [_ w764]
                tunnel: w752 -> [w760 w763]
                tunnel: [w760 w762] -> w751
                tunnel: w741 -> [_ w761]
                frame False {
                }
                frame True {
                  n299 = call "CleanupTraces.vi"("Baseline Rate"=w761, "Spacing"=w765, "decimating factor"=w764, "Traces in"=w763) -> ("Traces out"=w762:waveform(dbl)[])  [unwired: 7 in]
                }
              }
              "Traces" <- w751
            }
          }
          n300 = global read "GlobalVars.vi" "Scanning"() -> (w719:bool)
        }
        n301 = call-dynamic "Configure PointScan.vi"("AODAcq in"=w550, "Save"=TRUE ("Save Volume"), "Store Raw"="Store Raw", "Points"=w524, "GridSize"=w529, "Reps"=w568, "error in (no error)"=w583, "Motion Points"=w523, "Motion Increment"=w522) -> ("AODAcq out"=w574:refnum<class "AODAcq.lvclass">, "error out"=w575:errorcluster)  [unwired: 5 in]
        n302 = Initialize Array "Cumulative AOD Motion Signal"(w514, w513) -> (w512:dbl[])
        n303 = call-dynamic "Read FPGA VI Reference.vi"("error in (no error)"=w575, "AODAcq in"=w574) -> ("error out"=w565:errorcluster, "FPGA VI Reference"=w515:T11, "AODAcq out"=w511:refnum<class "AODAcq.lvclass">)  [unwired: 7 in]
        n304 = call-dynamic "Start.vi"("error in (no error)"=w565, "AODAcq in"=w511) -> ("error out"=w563:errorcluster, "AODAcq out"=w564:refnum<class "AODAcq.lvclass">)  [unwired: 8 in]
        n305 = call-dynamic "Read Recording File.vi"("error in (no error)"=w563, "AcquistionObject in"=w564) -> ("error out"=w558:errorcluster, "Recording File"=w562:path, "AcquistionObject out"=w510:refnum<class "AODAcq.lvclass">)  [unwired: 7 in]
        n306 = local write "Recording File"(w562) -> ()
        n307 = call-dynamic "Read Loop.vi"("error in (no error)"=w558, "ReadElements"=w577, "Queues"=w576, "AODAcq in"=w510) -> ("error out"=w508:errorcluster, "AODAcq out"=w509:refnum<class "AODAcq.lvclass">)  [unwired: 6 in]
        n308 = To Long Integer(number=w536) -> (32bit integer=w535:i32[][])
        n309 = while "Detect and Write Motor Position Information" {
          tunnel: w510 -> [w599]
          shift-right: [w597] -> _
          shift-left: w516 -> [w598]
          tunnel: w515 -> [w596]
          shift-right: [w594] -> _
          shift-left: w512 -> [w595]
          tunnel: w507 -> [w592]
          shift-right: [w587] -> _
          shift-left: 0 -> [w588]
          stop <- w600 continue-if-true
          n310 = Get Queue Status(queue=w592) -> (# elements in queue=→"Elements in Data Queue":i32)  [unwired: 2 in, 7 out]
          n311 = Dequeue Element(queue=w592, timeout in ms (-1)=10) -> (element=w589:T6, timed out?=w585:bool)  [unwired: 1 in, 2 out]
          n312 = local read "Motion Analysis"() -> (w586:bool)
          n313 = Not(x=w585) -> (.not. x?=w584:bool)
          n314 = And(x=w584, y=w586) -> (x .and. y?=w590:bool)
          n315 = case shown="True" w590 {
            tunnel: w599 -> [_ w641]
            tunnel: w598 -> [w603 w640]
            tunnel: [w603 w639] -> w597
            tunnel: w596 -> [_ w638]
            tunnel: w595 -> [w602 w637]
            tunnel: [w602 w636] -> w594
            tunnel: w592 -> [_ w618]
            tunnel: w589 -> [_ w615]
            tunnel: w588 -> [w601 w614]
            tunnel: [w601 w612] -> w587
            frame False {
            }
            frame True {
              n316 = Increment(x=w614) -> (x+1=w612:i32)
              n317 = global read "GlobalVars.vi" "Sampling Interval (sec)"() -> (w607:dbl)
              n318 = Bundle By Name(cluster=T10 {"Restarted"=FALSE, "Enable Calibration"=FALSE, "Position Shift Limit (Microns)"=3.0, "Frame Num"=0.0, "Sampling Interval"=0.0, "Analyze Nth Frames"=1} ("Params"), "Restarted"=FALSE, "Enable Calibration"="Enable Calibration", "Position Shift Limit (Microns)"="Position Shift Limit (Microns)", "Frame Num"=w612, "Sampling Interval"=w607, "Analyze Nth Frames"="Analyze Nth Frames") -> (w606:T10)
              n319 = call "RunDuringExperiment1.vi"("Params"=w606, "Motion Data In"=w615) -> ("Motion Computation Error"=w605:errorcluster, "Shifts Out"=w625:T12)  [unwired: 7 in, 1 out]
              n320 = Unbundle By Name(w625) -> ("X"=→"X1":waveform(dbl), "Y"=→"Y1":waveform(dbl), "Z"=→"Z1":waveform(dbl), "Out of Limits"=→"Out of Limits":bool, "Motion Detection Error"=→"Motion Detection Error":bool, "Flush Queue"=w619:i32, "Movement Signal"=w616:dbl[], "Movement Detection Time"=w617:dbl)
              n321 = flat-sequence {
                tunnel: [w644] -> w629
                tunnel: [w643] -> w627
                tunnel: w605 -> [w642]
                tunnel: [w642] -> w604
                frame #0 {
                  n322 = global read "GlobalVars.vi" "TargetPositionUpdateTime"() -> (w643:dbl)
                  n323 = Get Date/Time In Seconds() -> (seconds since 1Jan1904=w645:timestamp)
                  n324 = To Double Precision Float(number=w645) -> (double precision float=w644:dbl)
                }
              }
              n325 = feedback #2(0.0 ("Double")) -> (w630:dbl)
              n326 = feedback-in #2(w617) -> ()
              n327 = case shown="1" w619 {
                tunnel: w618 -> [_ w646]
                frame 0, Default {
                }
                frame 1 {
                  n328 = Flush Queue(queue=w646) -> ()  [unwired: 1 in, 3 out]
                }
              }
              n329 = global write "GlobalVars.vi" "MovementSignal"(w616) -> ()
              n330 = global write "GlobalVars.vi" "MovementDetectionTime"(w617) -> ()
              n331 = case shown="Error" w604 {
                selector: w604 -> [_ w648]
                frame No Error {
                }
                frame Error {
                  n332 = Unbundle By Name(w648) -> ("source"=w647:string)
                  n333 = One Button Dialog(message=w647) -> ()  [unwired: 1 in, 1 out]
                }
              }
              n334 = Subtract(x=w629, y=w627) -> (x-y=w635:dbl)
              n335 = Not Equal?(x=w617, y=w630) -> (x != y?=w631:bool)
              n336 = Greater?(x=w635, y="Motor Refractory Time") -> (0:w634:bool)
              n337 = And(x=w631, y=w634) -> (x .and. y?=w633:bool)
              n338 = case shown="True" "Motion Tracking" {
                tunnel: w641 -> [w651 w666]
                tunnel: w640 -> [w652 w669]
                tunnel: [w650 w667] -> w639
                tunnel: w616 -> [w653 w670]
                tunnel: w638 -> [_ w668]
                tunnel: w637 -> [w654 w665]
                tunnel: [w654 w664] -> w636
                tunnel: w633 -> [w649 w663]
                frame False {
                  n339 = case shown="True" w649 {
                    tunnel: w653 -> [_ w656]
                    tunnel: w652 -> [w655 w662]
                    tunnel: w651 -> [_ w660]
                    tunnel: [w655 w658] -> w650
                    frame False {
                    }
                    frame True {
                      n340 = shared-variable "My Computer\\SutterShared.lvlib\\TargetPosition"(w656) -> ()  [unwired: 1 in, 1 out]
                      n341 = Add(x=w662, y=w656) -> (x+y=w658:dbl[])
                      n342 = Get Date/Time In Seconds() -> (seconds since 1Jan1904=w661:timestamp)
                      n343 = To Double Precision Float(number=w661) -> (double precision float=w657:dbl)
                      n344 = global write "GlobalVars.vi" "TargetPositionUpdateTime"(w657) -> ()
                      n345 = Build Array (concatenate)(w657, w656) -> (w659:dbl[])
                      n346 = call "WriteMotorCorrectionData.vi"("Motion Correction Data"=w659, "AODAcq in"=w660) -> ()  [unwired: 8 in, 2 out]
                    }
                  }
                }
                frame True {
                  n347 = case shown="True" w663 {
                    tunnel: w670 -> [_ w673]
                    tunnel: w669 -> [w671 w676]
                    tunnel: w668 -> [_ w682]
                    tunnel: [w671 w675] -> w667
                    tunnel: w666 -> [_ w679]
                    tunnel: w665 -> [w672 w674]
                    tunnel: [w672 w677] -> w664
                    frame False {
                    }
                    frame True {
                      n348 = Add(x=w674, y=w673) -> (x+y=w678:dbl[])
                      n349 = Absolute Value(x=w678) -> (abs(x)=w680:dbl[])
                      n350 = Greater?(x=w680, y="Motor Correction Threshold") -> (0:w684:bool[])
                      n351 = Or Array Elements(Boolean array=w684) -> (logical OR=w683:bool)
                      n352 = case "If above threshold, move motors and zero all aod cumulative offsets" shown="True" w683 {
                        tunnel: w678 -> [w693 w704]
                        tunnel: w682 -> [w694 w708]
                        tunnel: [w693 w700] -> w677
                        tunnel: w679 -> [_ w709]
                        tunnel: w676 -> [w692 w705]
                        tunnel: [w692 w703] -> w675
                        tunnel: w674 -> [_ w698]
                        tunnel: w673 -> [w691 _]
                        frame False {
                          n353 = local read "Scan Settings (um)"() -> (w690:T2)
                          n354 = local read "Scan Settings"() -> (w689:T2)
                          n355 = call "MicronsToSetting.vi"("Scan Settings"=w689, "Scan Settings (um)"=w690, "Microns (X,Y,Z)"=w691) -> ("Setting"=w688:i32[])  [unwired: 8 in]
                          n356 = Index Array(array=w688, index #1=0 ("index"), index #2=0 ("index"), index #3=0 ("index")) -> (element #1=w687:i32, element #2=w686:i32, element #3=w685:i32)
                          n357 = xnode "Read/Write Control"("FPGA VI Reference In"=w694, "InOffset.X"=w687, "InOffset.Y"=w686, "InOffset.Z"=w685) -> ()  [unwired: 1 in, 2 out]
                        }
                        frame True {
                          w702 = 0 ("InOffset.X")
                          n358 = shared-variable "My Computer\\SutterShared.lvlib\\TargetPosition"(w704) -> ()  [unwired: 1 in, 1 out]
                          n359 = Add(x=w705, y=w704) -> (x+y=w703:dbl[])
                          n360 = xnode "Read/Write Control"("FPGA VI Reference In"=w708, "InOffset.X"=w702, "InOffset.Y"=w702, "InOffset.Z"=w702) -> ()  [unwired: 1 in, 2 out]
                          n361 = Get Date/Time In Seconds() -> (seconds since 1Jan1904=w707:timestamp)
                          n362 = To Double Precision Float(number=w707) -> (double precision float=w701:dbl)
                          n363 = Build Array (concatenate)(w701, w704) -> (w706:dbl[])
                          n364 = global write "GlobalVars.vi" "TargetPositionUpdateTime"(w701) -> ()
                          n365 = call "WriteMotorCorrectionData.vi"("Motion Correction Data"=w706, "AODAcq in"=w709) -> ()  [unwired: 8 in, 2 out]
                          n366 = Multiply(x=0.0, y=w698) -> (x*y=w700:dbl[])
                        }
                      }
                    }
                  }
                }
              }
            }
          }
          n367 = global read "GlobalVars.vi" "Scanning"() -> (w600:bool)
        }
        n368 = flat-sequence {
          tunnel: w508 -> [w776]
          tunnel: [w776] -> w533
          frame #0 {
            n369 = local write "Finished"(TRUE ("Finished")) -> ()
          }
        }
        n370 = while {
          tunnel: w541 -> [_]
          tunnel: w538 -> [w803]
          tunnel: w539 -> [_]
          tunnel: w515 -> [w824]
          tunnel: w573 -> [w820]
          tunnel: w572 -> [_]
          tunnel: w571 -> [w810]
          tunnel: w507 -> [w816]
          tunnel: w523 -> [w808]
          tunnel: w544 -> [w809]
          shift-right: [w804] -> _
          shift-left: 0 -> [w805]
          tunnel: w542 -> [w806]
          tunnel: w535 -> [w792]
          i -> [w819]
          stop <- w813 stop-if-true
          w795 = 1000 ("length")
          n371 = Dequeue Element(queue=w820, timeout in ms (-1)=w803) -> (element=w815:waveform(i32)[])  [unwired: 1 in, 3 out]
          n372 = Square(x=w810) -> (x^2=w807:u16)
          n373 = local read "Finished"() -> (w817:bool)
          n374 = shared-variable "My Computer\\AODAcq.lvclass\\ScanFraction"() -> (w781:dbl)  [unwired: 1 in, 1 out]
          "ScanProgress" <- w781
          n375 = shared-variable "My Computer\\AODAcq.lvclass\\ReadFraction"() -> (w821:dbl)  [unwired: 1 in, 1 out]
          n376 = Multiply(x=w805, y=w795) -> (x*y=w797:i32)
          n377 = Divide(x=w808, y=w807) -> (x/y=w802:dbl)
          n378 = xnode "Read/Write Control"("FPGA VI Reference In"=w824, "Control.Abort"="Abort") -> ()  [unwired: 1 in, 2 out]
          n379 = Array Subset(array=w806, index (row)=w797, length (row)=w795) -> (w796:dbl[][])  [unwired: 2 in]
          n380 = Divide(x=w802, y=2.0) -> (x/y=w800:dbl)
          n381 = Not Equal To 0?(x=w819) -> (x != 0?=w818:bool)
          n382 = Greater?(x=w781, y="Onset (fraction)") -> (0:w783:bool)
          n383 = Greater?(x=w781, y="Offset (fraction)") -> (0:w777:bool)
          n384 = Round Toward +Infinity(x=w800) -> (ceil(x): smallest int >= x=w799:dbl)
          n385 = And(x=w817, y=w818) -> (x .and. y?=w813:bool)
          n386 = Reshape Array(w796, w795) -> (w794:dbl[])
          n387 = local write "Progress"(w821) -> ()
          n388 = And(x="Auto Recentering", y=w783) -> (x .and. y?=w782:bool)
          n389 = And(x="Auto Recentering", y=w777) -> (x .and. y?=w779:bool)
          n390 = To Long Integer(number=w794) -> (32bit integer=w793:i32[])
          n391 = Decrement(x="Motion Channel To Analyze") -> (x-1=w811:i32)
          n392 = Decrement(x=w799) -> (x-1=w798:dbl)
          n393 = Not(x=w813) -> (.not. x?=w814:bool)
          n394 = Index Array(array=w815, index=w811) -> (element=w822:waveform(i32))
          n395 = case shown="True" w782 {
            frame False {
            }
            frame True {
              n396 = shared-variable "My Computer\\BehaviorShared.lvlib\\PauseBehavior"(TRUE ("PauseBehavior")) -> ()  [unwired: 1 in, 1 out]
            }
          }
          n397 = case shown="True" w779 {
            frame False {
            }
            frame True {
              n398 = shared-variable "My Computer\\BehaviorShared.lvlib\\PauseBehavior"(FALSE ("PauseBehavior")) -> ()  [unwired: 1 in, 1 out]
            }
          }
          n399 = global write "GlobalVars.vi" "Scanning"(w814) -> ()
          n400 = Unbundle By Name(w822) -> ("Y"=w791:i32[])
          n401 = call "Motion FIFO.vi"("Packet Length"=w808, "Data"=w791, "Motion FIFO"=w809) -> ("Number of Packets"=w788:i32, "Array"=w790:i32[])  [unwired: 7 in]
          n402 = Select(t=w793, s="Simulated Motion Signal", f=w790) -> (s? t:f=w789:i32[])
          n403 = Select(t=1, s="Simulated Motion Signal", f=w788) -> (s? t:f=w786:i32)
          n404 = for {
            N: w786 -> [_]
            tunnel: w816 -> [w854]
            tunnel: w810 -> [w839]
            tunnel: w789 -> [w853]
            tunnel: w808 -> [w850]
            tunnel: w807 -> [_]
            tunnel: w805 -> [w848]
            tunnel: w805 -> [w846]
            tunnel: [w845] -> w804
            tunnel: w798 -> [w842]
            tunnel: w792 -> [w836]
            tunnel: "Simulated Motion Signal" -> [w835]
            i -> [w847]
            w841 = 1 ("length")
            n405 = Multiply(x=w850, y=w847) -> (x*y=w852:i32)
            n406 = Array Subset "Select Packet"(array=w853, index=w852, length=w850) -> (w830:i32[])
            n407 = local read "Number of Motion Volumes"() -> (w832:i32)
            n408 = Array Size(array=w830) -> (size(s)=w833:i32)
            n409 = Divide(x=w833, y=w832) -> (x/y=w827:dbl)
            n410 = Array Subset "Select First Motion Volume"(array=w830, index=0, length=w827) -> (w828:i32[])
            n411 = Array Size(array=w828) -> (size(s)=w829:i32)
            n412 = Reshape Array(w828, w839, w839, w839) -> (w843:i32[][][])
            n413 = Array Subset(array=w843, index (dim 2)=w842, length (dim 2)=w841) -> (w844:i32[][][])  [unwired: 4 in]
            n414 = Array Subset(array=w843, index (dim 0)=w842, length (dim 0)=w841) -> (w840:i32[][][])  [unwired: 4 in]
            n415 = Reshape Array(w828, w829, 1 ("dimension size")) -> (w849:i32[][])
            n416 = case shown="True" "Motion Analysis" {
              tunnel: w854 -> [_ w890]
              tunnel: w849 -> [_ w885]
              tunnel: w839 -> [_ w886]
              tunnel: w848 -> [_ w881]
              tunnel: w847 -> [_ w880]
              tunnel: w846 -> [w859 w876]
              tunnel: [w859 w875] -> w845
              tunnel: w836 -> [_ w872]
              tunnel: w835 -> [_ w871]
              tunnel: w827 -> [_ w865]
              frame False {
                n417 = disable-structure shown="Disabled" {
                  frame Disabled {
                    n418 = global read "GlobalVars.vi" "VI Open"() -> (w860:bool)
                    n419 = case shown="True" w860 {
                      frame False {
                      }
                      frame True {
                        n420 = global write "GlobalVars.vi" "VI Open"(FALSE ("VI Open")) -> ()
                        n421 = vi-ref "RunDuringExperiment.vi"() -> (w861:refnum<vi>)
                        n422 = invoke on="Invoke Node" class="VI" method="Abort VI"(reference=w861) -> (reference out=w863:refnum<vi>)  [unwired: 2 in, 2 out]
                        n423 = invoke class="VI" method="FP.Close"(reference=w863) -> ()  [unwired: 2 in, 3 out]
                      }
                    }
                  }
                  frame Enabled {
                  }
                }
              }
              frame True {
                n424 = Increment "Loop Counter"(x=w876) -> (x+1=w875:i32)
                n425 = disable-structure shown="Disabled" {
                  frame Disabled {
                    n426 = global read "GlobalVars.vi" "VI Open"() -> (w891:bool)
                    n427 = case shown="False" w891 {
                      frame False {
                        n428 = vi-ref "RunDuringExperiment.vi"() -> (w892:refnum<vi>)
                        n429 = invoke on="Invoke Node" class="VI" method="FP.Open"(reference=w892) -> (reference out=w895:refnum<vi>)  [unwired: 4 in, 4 out]
                        n430 = invoke class="VI" method="Run VI"(reference=w895, "Wait until done"=FALSE ("Wait Until Done"), "Auto Dispose Ref"=TRUE ("Auto Dispose Reference")) -> ()  [unwired: 2 in, 5 out]
                      }
                      frame True {
                      }
                    }
                  }
                  frame Enabled {
                  }
                }
                n431 = Equal To 0?(x=w881) -> (x = 0?=w878:bool)
                n432 = Equal To 0?(x=w880) -> (x = 0?=w879:bool)
                n433 = And(x=w879, y=w878) -> (x .and. y?=w877:bool)
                n434 = local read "X-Y Motion Points"() -> (w870:i32[][])
                n435 = local read "Y-Z Motion Points"() -> (w867:i32[][])
                n436 = Array Subset(array=w870, index (row)=0 ("index"), length (row)=w865) -> (w868:i32[][])  [unwired: 2 in]
                n437 = Array Subset(array=w867, index (row)=0 ("index"), length (row)=w865) -> (w864:i32[][])  [unwired: 2 in]
                n438 = local read "Scan Settings (um)"() -> (w888:T2)
                n439 = local read "Scan Settings"() -> (w889:T2)
                n440 = Insert Into Array(array=w868, new element=w864) -> (w874:i32[][])  [unwired: 2 in]
                n441 = Select(t=w872, s=w871, f=w874) -> (s? t:f=w873:i32[][])
                n442 = Cluster To Array(cluster=w888) -> (array=w883:i32[])
                n443 = Cluster To Array(cluster=w889) -> (array=w884:i32[])
                n444 = Bundle By Name(cluster=T6 {"gridsize"=0, "data"=[], "coordinates"=[], "settings"=[], "settings_um"=[], "needsreference"=FALSE}, "gridsize"=w886, "data"=w885, "coordinates"=w873, "settings"=w884, "settings_um"=w883, "needsreference"=w877) -> (w882:T6)
                n445 = Lossy Enqueue Element(queue=w890, element=w882) -> ()  [unwired: 1 in, 4 out]
              }
            }
            n446 = Reshape Array(w844, w839, w839) -> (w837:i32[][])
            n447 = Reshape Array(w840, w839, w839) -> (w838:i32[][])
            n448 = Insert Into Array(array=w837, new element=w838) -> (w851:i32[][])  [unwired: 2 in]
            n449 = local read "Motion Ch1"() -> (w857:T5)
            n450 = To Single Precision Float(number=w851) -> (single precision float=w856:sgl[][])
            n451 = call "IMAQ ArrayToImage"("Image Pixels (Float)"=w856, "Image"=w857) -> ("Image Out"=w858:T5)  [unwired: 8 in, 1 out]
            n452 = local write "Motion Ch1"(w858) -> ()
          }
        }
      }
      frame 4 {
        n453 = call-dynamic "Reset.vi"("error in (no error)"=w898, "AODAcq in"=w899) -> ("error out"=w897:errorcluster, "AODAcq out"=w896:refnum<class "AODAcq.lvclass">)  [unwired: 8 in]
        n454 = call-dynamic "Read FPGA VI Reference.vi"("error in (no error)"=w897, "AODAcq in"=w896) -> ("error out"=w905:errorcluster, "FPGA VI Reference"=w906:T11, "AODAcq out"=w904:refnum<class "AODAcq.lvclass">)  [unwired: 7 in]
        n455 = flat-sequence {
          tunnel: w906 -> [w909]
          tunnel: w905 -> [w907]
          tunnel: w904 -> [w908]
          tunnel: [w908] -> w901
          tunnel: [w907] -> w900
          tunnel: [w911] -> w902
          tunnel: [w910] -> w903
          tunnel: w901 -> [w913]
          tunnel: w900 -> [w912]
          frame #0 {
            n456 = call "SweepSettings.vi"("FPGA VI Reference Out"=w909) -> ()  [unwired: 11 in]
          }
          frame #1 {
            n457 = call-dynamic "GetStatus.vi"("error in (no error)"=w912, "AODAcq in"=w913) -> ("error out"=w911:errorcluster, "AODAcq out"=w910:refnum<class "AODAcq.lvclass">)  [unwired: 7 in, 1 out]
          }
        }
      }
      frame 8 {
        n458 = Unbundle(w924) -> ("queue out"=w918:refnum<queue>)  [unwired: 3 out]
        n459 = local write "Ephys Acq"(FALSE ("Ephys")) -> ()
        n460 = local write "Ephys"(TRUE ("Ephys")) -> ()
        n461 = local write "Tab Control"(enum32{"Setup", "Volume", "Traces", "Motion"}."Traces" ("Tab Control")) -> ()
        n462 = call "DAQ Assistant"() -> ("task out"=w925:refnum<k21>, "error out"=w920:errorcluster)  [unwired: 16 in, 2 out]
        n463 = while {
          tunnel: w925 -> [w934]
          tunnel: w918 -> [w933]
          tunnel: [w932] -> w923
          tunnel: w920 -> [w931]
          tunnel: [w929] -> w919
          tunnel: [FALSE ("Ephys")] -> w915
          stop <- w935 stop-if-true
          n464 = call-poly <vilib>:"DAQmx Read.vi"("task/channels in"=w934, "error in"=w931) -> ("task out"=w932:refnum<k21>, "data"=w927:waveform(dbl), "error out"=w930:errorcluster)  [unwired: 11 in]
          "Waveform Chart" <- w927
          n465 = Build Array(w927) -> (w926:waveform(dbl)[])
          n466 = Enqueue Element(queue=w933, element=w926, error in (no error)=w930) -> (error out=w929:errorcluster)  [unwired: 1 in, 2 out]
          n467 = local read "Abort"() -> (w935:bool)
        }
        "Ephys" <- w915
        n468 = call <vilib>:"DAQmx Clear Task.vi"("task in"=w923, "error in"=w919) -> ("error out"=w921:errorcluster)  [unwired: 13 in]
      }
    }
    n469 = call <vilib>:"Release Semaphore.vi"("error in (no error)"=w258, "semaphore"=w259) -> ()  [unwired: 4 in, 2 out]
    n470 = call-dynamic "Stop.vi"("error in (no error)"=w264, "AODAcq in"=w266) -> ("error out"=w263:errorcluster, "AODAcq out"=w265:refnum<class "AODAcq.lvclass">)  [unwired: 8 in]
    "AODAcq out" <- w265
    n471 = call-dynamic "Read FPGA VI Reference.vi"("error in (no error)"=w263, "AODAcq in"=w265) -> ("error out"=w269:errorcluster, "FPGA VI Reference"=w270:T11)  [unwired: 7 in, 1 out]
    n472 = xnode "Read/Write Control"("FPGA VI Reference In"=w270, "error in"=w269) -> ("error out"=w268:errorcluster, "Control.Abort"=w271:bool)  [unwired: 1 out]
    n473 = while {
      tunnel: w268 -> [w307]
      tunnel: [w308] -> w273
      tunnel: [w307] -> w272
      stop <- TRUE stop-if-true
      n474 = local write "Finished"(FALSE ("Finished")) -> ()
      n475 = local read "Selection"() -> (w308:u32)
    }
    n476 = case shown="2" w273 {
      tunnel: w272 -> [w310 w316 w333]
      tunnel: [w310 w315 w332] -> w280
      tunnel: w271 -> [_ w311 w335]
      frame 0, Default {
        w309 = FALSE ("ForceVolumeScan")
        n477 = local write "ForcePointScan"(w309) -> ()
        n478 = local write "ForceVolumeScan"(w309) -> ()
      }
      frame 2 {
        n479 = local read "Auto Recentering"() -> (w314:bool)
        n480 = Not(x=w311) -> (.not. x?=w313:bool)
        n481 = And(x=w314, y=w313) -> (x .and. y?=w312:bool)
        n482 = case shown="True" w312 {
          tunnel: w316 -> [w318 w331]
          tunnel: [w318 w331] -> w315
          frame False {
            w317 = FALSE ("ForceVolumeScan")
            n483 = local write "ForcePointScan"(w317) -> ()
            n484 = local write "ForceVolumeScan"(w317) -> ()
          }
          frame True {
            n485 = local write "ForceVolumeScan"(TRUE ("ForceVolumeScan")) -> ()
            n486 = local write "ForcePointScan"(FALSE ("ForcePointScan")) -> ()
            n487 = local read "Scan Settings (um) Saved"() -> (w327:T2)
            n488 = local read "Scan Settings Saved"() -> (w322:T2)
            n489 = Bundle By Name(cluster=w327, "XNum"="XNum", "YNum"="YNum") -> (w328:T2)
            n490 = Unbundle By Name(w327) -> ("XNum"=w326:i32, "YNum"=w325:i32)
            n491 = Bundle By Name(cluster=w322, "XNum"="XNum", "YNum"="YNum") -> (w319:T2)
            n492 = Divide(x=w326, y="XNum") -> (x/y=→"x_scale":dbl)
            n493 = Divide(x=w325, y="YNum") -> (x/y=→"y_scale":dbl)
            n494 = local write "Scan Settings (um)"(w328) -> ()
            n495 = local write "Scan Settings"(w319) -> ()
          }
        }
      }
      frame 1 {
        n496 = local read "ForceVolumeScan"() -> (w334:bool)
        n497 = Not(x=w335) -> (.not. x?=w336:bool)
        n498 = And(x=w334, y=w336) -> (x .and. y?=w337:bool)
        n499 = case shown="False" w337 {
          tunnel: w335 -> [w340 _]
          tunnel: w334 -> [w339 _]
          tunnel: w333 -> [w338 w346]
          tunnel: [w338 w345] -> w332
          frame False {
            n500 = case shown="True" w340 {
              tunnel: w339 -> [_ w342]
              frame False {
              }
              frame True {
                n501 = case shown="True" w342 {
                  frame False {
                  }
                  frame True {
                    n502 = local write "ForceVolumeScan"(FALSE ("ForceVolumeScan")) -> ()
                    n503 = local read "Scan Settings (um) Saved"() -> (w343:T2)
                    n504 = local write "Scan Settings (um)"(w343) -> ()
                  }
                }
              }
            }
            n505 = local write "ForcePointScan"(FALSE ("ForcePointScan")) -> ()
          }
          frame True {
            n506 = stacked-sequence {
              tunnel: w346 -> [w364 _ _ _ _]
              tunnel: [w363 _ _ _ _] -> w345
              frame #0 {
                # "Assumes same 'Z\" resolution"
                n507 = local write "EventDone"(FALSE ("EventDone")) -> ()
                n508 = local read "Scan Settings (um) Saved"() -> (w365:T2)
                n509 = local read "Scan Settings (um)"() -> (w375:T2)
                n510 = Unbundle(w365) -> ("XStart"=w366:i32, "XEnd"=w367:i32, "XNum"=w368:i32, "YStart"=w369:i32, "YEnd"=w370:i32, "YNum"=w371:i32, "ZStart"=w372:i32, "ZEnd"=w373:i32, "ZNum"=w374:i32)
                n511 = Unbundle(w375) -> ("XStart"=w376:i32, "XEnd"=w377:i32, "XNum"=w378:i32, "YStart"=w379:i32, "YEnd"=w380:i32, "YNum"=w381:i32, "ZStart"=w382:i32, "ZEnd"=w383:i32, "ZNum"=w384:i32)
                n512 = local read "VolData"() -> (w385:i32[][])
                n513 = Build Array(w366, w367, w368, w369, w370, w371, w372, w373, w374) -> (w362:i32[])
                n514 = Build Array(w376, w377, w378, w379, w380, w381, w382, w383, w384) -> (w361:i32[])
                n515 = script code="x = linspace(settings(1),settings(2),settings(3));\ny = linspace(settings(4),settings(5),settings(6));\nz = linspace(settings(7),settings(8),settings(9));\n\nox = linspace(osettings(1),osettings(2),osettings(3));\noy = linspace(osettings(4),osettings(5),osettings(6));\noz = linspace(osettings(7),osettings(8),osettings(9));\n\nstack = stack(1,:);\nstack = reshape(stack,numel(y),numel(x),numel(z));\n\nvolout = zeros( numel(oy), numel(ox), numel(oz)) ;\nfor ii=1:size(stack,3)\n    volout(:,:,ii) = imresize(squeeze(stack(:,:,ii)), [size(volout,1) size(volout,2)], 'nearest') ;\nend ;\n\nvolout = reshape(volout, 1, numel(oy)*numel(ox)*numel(oz)) ;"("??"=w364, "stack"=w385, "settings"=w361, "osettings"=w362) -> ("??"=w363:errorcluster, "volout"=w358:dbl[][])
                n516 = local read "Scan Settings Saved"() -> (w356:T2)
                n517 = local read "Contrast"() -> (w352:dbl)
                n518 = local read "Section"() -> (w348:dbl)
                n519 = To Long Integer(number=w358) -> (32bit integer=w357:i32[][])
                n520 = local write "VolData"(w357) -> ()
                n521 = global write "GlobalVars.vi" "VolumeData"(w357) -> ()
                n522 = local read "ImCh1"() -> (w355:T5)
                n523 = local read "ImCh2"() -> (w354:T5)
                n524 = local read "Offset"() -> (w353:dbl)
                n525 = call "Convert to Dynamic Data2"("2D Array"=w357) -> ("Dynamic Data Type"=w359:dynamicdata)  [unwired: 3 in]
                n526 = local read "Mirror Ch1 Display"() -> (w350:bool)
                n527 = call "UpdateStack.vi"("Contrast"=w352, "Scan Settings"=w356, "Offset"=w353, "Section"=w348, "ImData"=w357, "Im2 2"=w354, "Im1 In"=w355) -> ("Im2 Out"=w360:T5, "Im1 Out"=w347:T5)  [unwired: 3 in]
                n528 = call "Create Histogram2"("Signal"=w359) -> ("Histogram"=w351:dynamicdata)  [unwired: 9 in, 1 out]
                n529 = local write "ImCh1"(w347) -> ()
                n530 = local write "Histogram"(w351) -> ()
                n531 = case shown="True" w350 {
                  tunnel: w347 -> [_ w389]
                  tunnel: [w387 w388] -> w349
                  tunnel: w360 -> [w387 w390]
                  frame False {
                  }
                  frame True {
                    n532 = call "IMAQ Copy"("Image Dst"=w390, "Image Src"=w389) -> ("Image Dst Out"=w388:T5)  [unwired: 4 in, 1 out]
                  }
                }
                n533 = local write "ImCh2"(w349) -> ()
              }
              frame #1 {
                n534 = local read "Scan Settings Saved"() -> (w391:T2)
                n535 = local read "Scan Settings (um) Saved"() -> (w392:T2)
                n536 = local write "Scan Settings"(w391) -> ()
                n537 = local write "Scan Settings (um)"(w392) -> ()
              }
              frame #2 {
                n538 = property on="Recenter" class="Bool (strict)"("Val(Sgnl)"=TRUE ("Value (Signaling)")) -> ()  [unwired: 2 in, 2 out]
              }
              frame #3 {
                n539 = while {
                  tunnel: [FALSE ("Value (Signaling)")] -> w394
                  stop <- w396 stop-if-true
                  n540 = local read "EventDone"() -> (w396:bool)
                }
                n541 = property on="Recenter" class="Bool (strict)"("Val(Sgnl)"=w394) -> ()  [unwired: 2 in, 2 out]
              }
              frame #4 {
                n542 = local write "ForceVolumeScan"(FALSE ("ForceVolumeScan")) -> ()
                n543 = local write "ForcePointScan"(TRUE ("ForcePointScan")) -> ()
                n544 = Wait (ms)(milliseconds to wait="Post Recentering Wait (ms)") -> ()  [unwired: 1 out]
              }
            }
          }
        }
      }
    }
    n545 = call <vilib>:"Simple Error Handler.vi"("error in (no error)"=w280) -> ()  [unwired: 4 in, 5 out]
    "Volume" <- "Volume Scan"
    "Scan" <- "Points Scan"
    "Numeric" <- w287
  }
  "Stopped" <- w18
  n546 = while {
    tunnel: w32 -> [w938]
    stop <- w937 stop-if-true
    n547 = local read "Tab Control"() -> (w936:enum32{"Setup", "Volume", "Traces", "Motion"})
    n548 = case shown="\"Traces\"" w936 {
      tunnel: w938 -> [_ w944]
      frame "Setup", Default {
        n549 = Wait (ms)(milliseconds to wait=u32 150) -> ()  [unwired: 1 out]
      }
      frame "Traces" {
        n550 = Dequeue Element(queue=w944, timeout in ms (-1)=500) -> (element=w941:waveform(dbl)[], timed out?=w940:bool, error out=w942:errorcluster)  [unwired: 1 in, 1 out]
        n551 = call <vilib>:"Clear Errors.vi"("error in (no error)"=w942) -> ()  [unwired: 5 in, 2 out]
        n552 = case shown="False" w940 {
          tunnel: w941 -> [w945 _]
          frame False {
            "Ephys Signals" <- w945
          }
          frame True {
          }
        }
      }
    }
    n553 = local read "Stopped"() -> (w937:bool)
  }
  n554 = case shown="True" w18 {
    tunnel: [errorcluster {"status"=FALSE, "code"=0, "source"=""} ("error out") w948] -> w19
    frame False {
    }
    frame True {
      n555 = global read "GlobalVars.vi" "VI Open"() -> (w947:bool)
      n556 = case shown="True" w947 {
        tunnel: [errorcluster {"status"=FALSE, "code"=0, "source"=""} ("error out") w953] -> w948
        frame False {
        }
        frame True {
          n557 = vi-ref "RunDuringExperiment.vi"() -> (w950:refnum<vi>)
          n558 = global write "GlobalVars.vi" "VI Open"(FALSE ("VI Open")) -> ()
          n559 = invoke on="Invoke Node" class="VI" method="Abort VI"(reference=w950) -> (reference out=w952:refnum<vi>)  [unwired: 2 in, 2 out]
          n560 = invoke class="VI" method="FP.Close"(reference=w952) -> (error out=w953:errorcluster)  [unwired: 2 in, 2 out]
        }
      }
    }
  }
  n561 = stacked-sequence {
    tunnel: w19 -> [_ w957]
    frame #0 {
      n562 = Wait Until Next ms Multiple(millisecond multiple=u32 500) -> ()  [unwired: 1 out]
    }
    frame #1 {
      n563 = disable-structure shown="Disabled" {
        disable-tunnel: w957 -> [w961 _]
        frame Disabled {
          n564 = global read "GlobalVars.vi" "MotionAnalysis"() -> (w959:refnum<queue>)
          n565 = local read "Motion FIFO"() -> (w960:refnum<queue>)
          n566 = Release Queue(queue=w959, error in (no error)=w961) -> (error out=w958:errorcluster)  [unwired: 1 in, 2 out]
          n567 = Release Queue(queue=w960, error in (no error)=w958) -> ()  [unwired: 1 in, 3 out]
        }
        frame Enabled {
        }
      }
      n568 = local read "Scan Settings Saved"() -> (w955:T2)
      n569 = local read "Scan Settings (um) Saved"() -> (w956:T2)
      n570 = local write "Scan Settings"(w955) -> ()
      n571 = local write "Scan Settings (um)"(w956) -> ()
    }
  }
  "Points_um" <- dbl[][] [] ("Points_um")
